vi "SignalViewer.vi"() -> ()   [LabVIEW 2014]
uses:
  <vilib>/Analysis/3filter.llb/Filter Passband Type.ctl
  <vilib>/Analysis/3filter.llb/Filter Structure Type.ctl
  <vilib>/event_ctls.llb/eventvkey.ctl
  <vilib>/Utility/miscctls.llb/LVPositionTypeDef.ctl
  <vilib>/Utility/miscctls.llb/LVKeyTypeDef.ctl
  <vilib>/imath/engines/lvmath/Plug In/_Char/NIMS_CH_character datatype.ctl
  <vilib>/Analysis/2dsp.llb/Decimate (single shot, DBL).vi
  <vilib>/Analysis/baseanly.llb/Mean (DBL).vi
  <vilib>/Analysis/3filter.llb/Savitzky-Golay Filter (DBL).vi
  <vilib>/Waveform/WDTOps.llb/WDT Waveform Duration DBL.vi
  <vilib>/Utility/file.llb/Write To Spreadsheet File (string).vi
  <vilib>/Utility/file.llb/Read From Spreadsheet File (string).vi
  <vilib>/Waveform/WDTOps.llb/WDT Get Waveform Time Array DBL.vi
  <vilib>/Waveform/WDTOps.llb/WDT Scale Delta t DBL.vi
  <vilib>/Waveform/WDTOps.llb/WDT Get Waveform Subset DBL.vi
  <vilib>/measure/matone.llb/Extract Single Tone Information 1 Chan.vi
  <vilib>/Analysis/3filter.llb/Zero Phase Filter (Cascade, DBL).vi
  <vilib>/addons/Time Frequency Analysis/Spectrogram.llb/TFA STFT Spectrogram (Waveform).vi
  <vilib>/addons/Time Frequency Analysis/_control.llb/TFA Configure Spectrogram Indicator (Predefined Color Table).vi
  <vilib>/addons/Time Series Analysis/Correlation and Spectral Analysis.llb/TSA Welch (Waveform).vi
  <vilib>/imath/engines/lvmath2/RunTimeEngine/Managers/WorkSpace/UID Generator.vi
  <vilib>/imath/engines/lvmath2/RunTimeEngine/BuiltInFunctions/win_hamming/NIMS_win_hamming.vi
  <vilib>/imath/engines/lvmath2/RunTimeEngine/ErrorHandling/NIMS_Error From Error Code.vi
  <vilib>/imath/engines/lvmath2/RunTimeEngine/BuiltInFunctions/coherence/NIMS_coherence().vi
  <instcachedir>/0/NIMS_coherence()_7638C21039694BA7B313C9663B018448.lvgen/NIMS_coherence()_7638C21039694BA7B313C9663B018448_000.vi
  <vilib>/imath/engines/lvmath2/RunTimeEngine/ErrorHandling/NIMS_Create Error From Enums.vi
  <vilib>/imath/engines/lvmath2/RunTimeEngine/IndexRead/NIMS M(S).vi
  <instcachedir>/0/NIMS M(S)_B826C018497E4940AE96BD27B540B6FB.lvgen/NIMS M(S)_B826C018497E4940AE96BD27B540B6FB_000.vi
  <vilib>/imathl/engines/lvmath/Functions/Error Handling/Create Error.vi
  <vilib>/imath/engines/lvmath2/RunTimeEngine/BuiltInFunctions/crosspsd/NIMS_crosspsd().vi
  <instcachedir>/0/NIMS_crosspsd()_8F170A66E657497C8ED809E1A8C589EF.lvgen/NIMS_crosspsd()_8F170A66E657497C8ED809E1A8C589EF_000.vi
  <vilib>/imath/engines/lvmath2/RunTimeEngine/RunTimeType/NIMS_RunTimeType_From StrictType (excl LVString).vi
  <instcachedir>/0/NIMS_RunTimeType_From StrictType (excl LVString)_15A5391EEA9C4AACB9955AC755B83D29.lvgen/NIMS_RunTimeType_From StrictType (excl LVString)_15A5391EEA9C4AACB9955AC755B83D29_000.vi
  <vilib>/imath/engines/lvmath2/RunTimeEngine/LocalVariableDefStatement/MC_LocalVariableDefStatement_Display.vi
  <vilib>/imath/engines/lvmath2/RunTimeEngine/BuiltInFunctions/conjugate/NIMS_conjugate(Complex).vi
  <instcachedir>/0/NIMS_conjugate(Complex)_151E186CA54B4853A0120BB0A667D86E.lvgen/NIMS_conjugate(Complex)_151E186CA54B4853A0120BB0A667D86E_001.vi
  <vilib>/imath/engines/lvmath2/RunTimeEngine/BuiltInFunctions/imag/NIMS_imag(Complex).vi
  <instcachedir>/0/NIMS_imag(Complex)_3180D40D00C843A49C2B33397F857BF3.lvgen/NIMS_imag(Complex)_3180D40D00C843A49C2B33397F857BF3_002.vi
  <vilib>/imath/engines/lvmath2/RunTimeEngine/BuiltInFunctions/angle/NIMS_angle.vi
  <instcachedir>/0/NIMS_angle_6DDAE2BD99E0421EB990B6436E94D88F.lvgen/NIMS_angle_6DDAE2BD99E0421EB990B6436E94D88F_002.vi
  <vilib>/imath/engines/lvmath2/RunTimeEngine/BuiltInFunctions/rad_to_deg/NIMS_rad_to_deg.vi
  <instcachedir>/0/NIMS_rad_to_deg_A39AFCDDC8C049FCADAAB7FC30B9F5AA.lvgen/NIMS_rad_to_deg_A39AFCDDC8C049FCADAAB7FC30B9F5AA_001.vi
  <vilib>/imath/engines/lvmath2/RunTimeEngine/BuiltInFunctions/unwrapphase/NIMS_unwrapphase(M,M,I32).vi
  <vilib>/imath/engines/lvmath2/RunTimeEngine/BuiltInFunctions/abs/NIMS_abs(signed).vi
  <instcachedir>/0/NIMS_abs(signed)_C4FCB8E6058B49B797C7C8D53CA5F6EC.lvgen/NIMS_abs(signed)_C4FCB8E6058B49B797C7C8D53CA5F6EC_006.vi
  <vilib>/imath/engines/lvmath2/RunTimeEngine/NodeEndStatement/NIMS_NodeEndStatement_Get Vector.vi
  <instcachedir>/0/NIMS_NodeEndStatement_Get Vector_00D1625602D843AD9D7EC134A9EC13A2.lvgen/NIMS_NodeEndStatement_Get Vector_00D1625602D843AD9D7EC134A9EC13A2_001.vi
  <vilib>/imath/engines/lvmath/Functions/Error Handling/MergeErrorsWrapper.vi
  <vilib>/imath/engines/lvmath2/RunTimeEngine/Managers/SymbolTable/Clear UID.vi
  <vilib>/imath/engines/lvmath2/RunTimeEngine/NodeEndStatement/NIMS_NodeEndStatement_Output.vi
  <instcachedir>/0/NIMS_NodeEndStatement_Output_53EC0D466D134D7ABD903AC30B43404B.lvgen/NIMS_NodeEndStatement_Output_53EC0D466D134D7ABD903AC30B43404B_001.vi
  <instcachedir>/0/NIMS_NodeEndStatement_Output_53EC0D466D134D7ABD903AC30B43404B.lvgen/NIMS_NodeEndStatement_Output_53EC0D466D134D7ABD903AC30B43404B_005.vi
  <vilib>/imath/engines/lvmath2/RunTimeEngine/ErrorHandling/NIMS_Finalize Error.vi
  <vilib>/imath/engines/lvmath2/RunTimeEngine/BuiltInFunctions/psd_welch/NIMS_psd_welch().vi
  <instcachedir>/0/NIMS_psd_welch()_5616DAC80B234F9987AA290C647A4538.lvgen/NIMS_psd_welch()_5616DAC80B234F9987AA290C647A4538_000.vi
  <vilib>/imath/engines/lvmath2/RunTimeEngine/IndexRead/NIMS V(S).vi
  <instcachedir>/0/NIMS V(S)_0488751826AF41519A22953C041130DC.lvgen/NIMS V(S)_0488751826AF41519A22953C041130DC_000.vi
  <vilib>/addons/_Advanced Signal Processing/NI_AdvSigProcTSA.lvlib
  <vilib>/Analysis/NI_AALBase.lvlib
  <vilib>/addons/_Advanced Signal Processing/NI_AdvSigProcTFA.lvlib
  <vilib>/measure/NI_MAPro.lvlib
  <vilib>/imath/engines/lvmath2/RunTimeEngine/Managers/SymbolTable/NIMS_WorkSpace.lvlib
  <vilib>/Analysis/NI_AALPro.lvlib
panel:
  out "listOfProfiles":path[](array[path])
  in  "write":bool
  in  "XY":bool
  in  "picker":i32(ring) items=["AllPlots", "13.06.17\\_0005#2_dt=2.40E-6orig", "13.06.17\\_0005#4_dt=2.40E-6orig", "13.06.17\\_0005#6_dt=2.40E-6orig", "13.06.17\\_0005#10_dt=2.40E-6orig"]
  in  "step, ms":dbl=1.0
  in  "howmany":u32=10 min=1
  in  "points":bool
  in  "clear":bool
  in  "scale fit":bool
  in  "path-name":bool=TRUE
  in  "show legend":bool
  in  "data info template":T1={"data path"="", "ADCintercadr_s"=1.0, "data info"={"use or not *.info.txt?"=0, "probe name"="NaN", "signal type"="NaN", "Unit"="NaN", "variable"="NaN", "attenuation factor"=1.0, "amplification factor"=1.0, "extracoef#1"=1.0, "extracoef#2"=1.0, "U cascade, kV"="NaN", "probe area, cm2"=1.0, "plasma, a.m.u."=1.0}, "channel_name"="", "channels_in_file"=0, "LastModified"=""}
  out "allinfos":T2(array[cluster])
  in  "0-color":u32(colorbox)=4456703
  in  "\"0\" line":bool
  in  "zero drift control":T3={"start zero, ms"=1.0, "duration of zero,ms"=1.0, "'0',\nms"=FALSE} {"start zero, ms" min=0.002400000058593751 max=49.996801220625024; "duration of zero,ms" min=0.002400000058593751 max=49.996801220625024}
  in  "autopen":cluster{"howmany":i16, "auto/man.":bool}={"howmany"=1, "auto/man."=FALSE} {"howmany" min=1}
  in  "show all":bool
  in  "cleararray":bool
  in  "regime":u16(ring) items=["data", "spectfilt", "preprocessed", "triple probe"]
  in  "open":bool
  in  "applyInfo":bool
  in  "setInfo":bool
  in  "writedat":bool
  out "spectrogram array":dbl[][][](array[numeric])
  in  "scalefit2":bool
  out "chan.in.files":i16[](array[numeric])
  in  "curs.":bool
  in  "curs.0":bool
  out "cursors":T4 {"Y1" format="%#.7f"; "X1" format="%#.7f"; "Y" format="%#.7f"; "X" format="%#.7f"}
  in  "EX":bool
  in  "width":i16 min=0 max=5 step=1
  in  "aver.\ncolor":u32(colorbox)=16711680
  in  "smooth":u16(ring) items=["origin"=0, "orig&med"=5, "orig-med"=6, "orig&poly"=1, "orig-poly"=3, "polynom"=2, "median"=4]
  in  "polyn.\norder":i32=1 min=1
  in  "wind.,\nms":dbl=1.0 min=0.004800000117187502 max=24.998400610312512
  out "nextfile":bool
  out "return pressed?":bool
  out "recalculate?":bool
  in  "tripleProbeSetting":T5={"Isat"=0, "Vfl"=0, "V+"=0, "a=1/ln2"=1.44, "Vfl*"=1.0, "[V+]*"=1.0, "Te*"=2.5, "/Rn(ohm)"=1.0, "/amplif"=1.0, "Spr, cm^2"=0.07, "plasma, a.m.u"=1.0, "Ne*10^x"=11.0} {"Ne*10^x" min=1.0 max=20.0 step=1.0; "V+" items=["14.06.17\\_0001=t0.000000-0.050000#2", "14.06.17\\_0001=t0.000000-0.050000#4", "14.06.17\\_0001=t0.000000-0.050000#6", "14.06.17\\_0002=t0.000000-0.050000#2", "14.06.17\\_0002=t0.000000-0.050000#4", "14.06.17\\_0002=t0.000000-0.050000#6", "14.06.17\\_0003=t0.000000-0.050000#2", "14.06.17\\_0003=t0.000000-0.050000#4", "14.06.17\\_0003=t0.000000-0.050000#6", "14.06.17\\_0004=t0.000000-0.050000#2", "14.06.17\\_0004=t0.000000-0.050000#4", "14.06.17\\_0004=t0.000000-0.050000#6", "14.06.17\\_0005=t0.000000-0.050000#2", "14.06.17\\_0005=t0.000000-0.050000#4", "14.06.17\\_0005=t0.000000-0.050000#6"]; "Vfl" items=["14.06.17\\_0001=t0.000000-0.050000#2", "14.06.17\\_0001=t0.000000-0.050000#4", "14.06.17\\_0001=t0.000000-0.050000#6", "14.06.17\\_0002=t0.000000-0.050000#2", "14.06.17\\_0002=t0.000000-0.050000#4", "14.06.17\\_0002=t0.000000-0.050000#6", "14.06.17\\_0003=t0.000000-0.050000#2", "14.06.17\\_0003=t0.000000-0.050000#4", "14.06.17\\_0003=t0.000000-0.050000#6", "14.06.17\\_0004=t0.000000-0.050000#2", "14.06.17\\_0004=t0.000000-0.050000#4", "14.06.17\\_0004=t0.000000-0.050000#6", "14.06.17\\_0005=t0.000000-0.050000#2", "14.06.17\\_0005=t0.000000-0.050000#4", "14.06.17\\_0005=t0.000000-0.050000#6"]; "Isat" items=["14.06.17\\_0001=t0.000000-0.050000#2", "14.06.17\\_0001=t0.000000-0.050000#4", "14.06.17\\_0001=t0.000000-0.050000#6", "14.06.17\\_0002=t0.000000-0.050000#2", "14.06.17\\_0002=t0.000000-0.050000#4", "14.06.17\\_0002=t0.000000-0.050000#6", "14.06.17\\_0003=t0.000000-0.050000#2", "14.06.17\\_0003=t0.000000-0.050000#4", "14.06.17\\_0003=t0.000000-0.050000#6", "14.06.17\\_0004=t0.000000-0.050000#2", "14.06.17\\_0004=t0.000000-0.050000#4", "14.06.17\\_0004=t0.000000-0.050000#6", "14.06.17\\_0005=t0.000000-0.050000#2", "14.06.17\\_0005=t0.000000-0.050000#4", "14.06.17\\_0005=t0.000000-0.050000#6"]}
  in  "inpcontrclaster":T6={"showwhat"={"total\nplots"=4, "show\nplots"=100, "show one/all"=FALSE, "ch#"=1, "visible\nplots"=4, "main loop\nwait, ms"=-1, "Y shift"=0.0, "txt rate,kHz"=625.0, "AxisX"=1, "X shift,ms"=0.0}, "inp.control"=[{"dataname"=0, "X-shift, ms"=0.0, "Y-shift"=0.0, "width"=0, "Color"=0, "visible"=TRUE, "multiplic."=1.0}, {"dataname"=0, "X-shift, ms"=0.0, "Y-shift"=0.0, "width"=0, "Color"=128, "visible"=TRUE, "multiplic."=1.0}, {"dataname"=0, "X-shift, ms"=0.0, "Y-shift"=0.0, "width"=0, "Color"=16711680, "visible"=TRUE, "multiplic."=1.0}, {"dataname"=0, "X-shift, ms"=0.0, "Y-shift"=0.0, "width"=0, "Color"=65280, "visible"=TRUE, "multiplic."=1.0}], "factor"=0, "average"=FALSE, "decimate"=FALSE} {"factor" min=1; "inp.control"."multiplic." format="%_6g"; "inp.control"."width" min=0 max=5 step=1; "inp.control"."Y-shift" format="%.6f"; "inp.control"."dataname" items=["***", "_0005#2\\13.06.17", "_0005#4\\13.06.17", "_0005#6\\13.06.17", "_0005#10\\13.06.17"]; "showwhat"."AxisX" items=["index", "time,s", "time,ms"]; "showwhat"."main loop\nwait, ms" min=-1 step=1; "showwhat"."visible\nplots" min=1 max=3; "showwhat"."ch#" min=0 max=4; "showwhat"."show\nplots" min=1; "showwhat"."total\nplots" min=1 max=3}
  in  "preproc.settings":T7={"select1"=0, "select2"=0, "FFT Window info"={"Window"=2, "Length"=128, "Overlap (%)"=50.0, "log/lin"=FALSE}, "dist.,cm"=0.3, "PowerScale 2D"=1.0, "Plot.Line Width"=3, "spectrogram\nsampling inf"={"time steps"=-1, "frequency bins"=512}, "dB on?"=FALSE, "spctrgr.color"=0, "spctrgrmWhich"=0, "autoscale"=TRUE, "max.freq,Hz"=0.0, "maxFreqSet"=FALSE} {"spctrgrmWhich" items=["14.06.17\\_0010=t0.000000-0.050000#2", "14.06.17\\_0010=t0.000000-0.050000#4", "14.06.17\\_0010=t0.000000-0.050000#6", "14.06.17\\_0010=t0.000000-0.050000#10"]; "spctrgr.color" items=["Rainbow", "Inverse gray", "Gray"]; "Plot.Line Width" max=5; "select2" items=["coherence", "crosspsd", "phase", "phaseDegrees", "Wavenum", "Flux(nv)"]; "PowerScale 2D" format="%#_6e"; "select1" items=["preproc.data", "crossfunct.", "autopsd", "spctrgrm"]; "FFT Window info"."Window" items=["None ", "Hanning", "Hamming", "Blackman-Harris", "Exact Blackman", "Blackman", "Flat Top", "4 Term B-Harris ", "7 Term B-Harris", "Low Sidelobe"]}
  out "triple probe":waveform(dbl)[](graph)
  out "spctrgrmClaster":T8 {"X" format="%#.6f"}
  out "scale info":variant
  out "observeddir":T9
  out "cut.filtered":waveform(dbl)[](graph)
  out "source":T10
  out "data cut":T11
  in  "spectr.filt.":enum32{"Page 1"}(tab)
  out "singletoneresult":waveform(dbl)(graph)
  in  "lin/log":u8(ring) items=["lin", "log"]
  in  "channel":i32(ring) items=["14.06.17\\_0010=t0.000000-0.050000#2", "14.06.17\\_0010=t0.000000-0.050000#4", "14.06.17\\_0010=t0.000000-0.050000#6", "14.06.17\\_0010=t0.000000-0.050000#10"]
  in  "singletonecontroll":T12={"advanced search"={"approx.freq."=-1.0, "search(+/-%)"=5.0}, "remove\ntone"=FALSE} {"advanced search"."search(+/-%)" format="%0.2p"; "advanced search"."approx.freq." format="%0.2p"}
  out "singletone":T13 {"det. phase (deg)" format="%.2p"; "detect.freq.,Hz" format="%.4e"; "detected ampl." format="%#.4e"}
  in  "bandstop":T16={"order"=4, "filter type"=enum."Bandstop", "filter structure option"=10, "apply\nfilter"=FALSE} {"filter structure option" items=["IIR 2nd Order"=0, "IIR 4th Order"=1, "Auto Select"=10]}
  in  "export mode":T17(ring)=enum."residual signal"
  in  "show":bool
  in  "time-freq. sampling info":cluster{"time steps":i32, "freq.bins":i32}={"time steps"=-1, "freq.bins"=1024}
  in  "spectrogam window info":cluster{"type":i32, "length":i32}={"type"=2, "length"=-1} {"type" items=["None ", "Hanning", "Hamming", "Blackman-Harris", "Exact Blackman", "Blackman", "Flat Top", "4 Term B-Harris ", "7 Term B-Harris", "Low Sidelobe", "Gaussian"]}
  in  "color table":u16(ring) items=["Rainbow", "Inverse gray", "Gray"]
  in  "fit":bool=TRUE
  in  "dB on?":bool
  out "PSD":cluster{"f0":dbl, "df":dbl, "S(f)":dbl[]}(graph)={"f0"=0.0, "df"=2441.40625, "S(f)"=[]}
  in  "window info":T18={"window"=2, "length"=64, "overlap (%)"=50.0} {"window" items=["None ", "Hanning", "Hamming", "Blackman-Harris", "Exact Blackman", "Blackman", "Flat Top", "4 Term B-Harris ", "7 Term B-Harris", "Low Sidelobe"]}
  in  "freq.bins":i32=1024
  out "Spectrogram":dbl[][](graph)
  in  "param.table":T19={"data info manual input sample"=[["11_00_19", "2", "VG1#1", "LP_biasing", "10.25", "1", "1", "162", "1", "5,6", "0.07", "1"], ["=", "4", "VG1#2", "LP_current", "10.25", "1", "1", "300", "1", "5,6", "0.07", "1"], ["11_00_44", "2", "VG1#1", "LP_biasing", "10.25", "1", "1", "162", "1", "5,6", "0.07", "1"], ["=", "4", "VG1#2", "LP_current", "10.25", "1", "1", "300", "1", "5,6", "0.07", "1"]], "data info manual input"=[["11", "7", "VG8", "V", "10.25", "1", "1", "", "", "", "0.049", "1"], ["=", "0", "VG8", "I", "10.25", "1", "1", "", "", "", "0.049", "1"], ["=", "10", "VG8", "V", "10.25", "1", "1", "", "", "", "0.049", "1"], ["=", "0", "VG8", "I", "10.25", "1", "1", "", "", "", "0.049", "1"]], "press after parram.input"=FALSE}
  out "data view":waveform(dbl)[](graph) caption="ADC data"
  # "Te=([V+]-[Vfl])*a"
  # "Vpl=Vfl+d*Te"
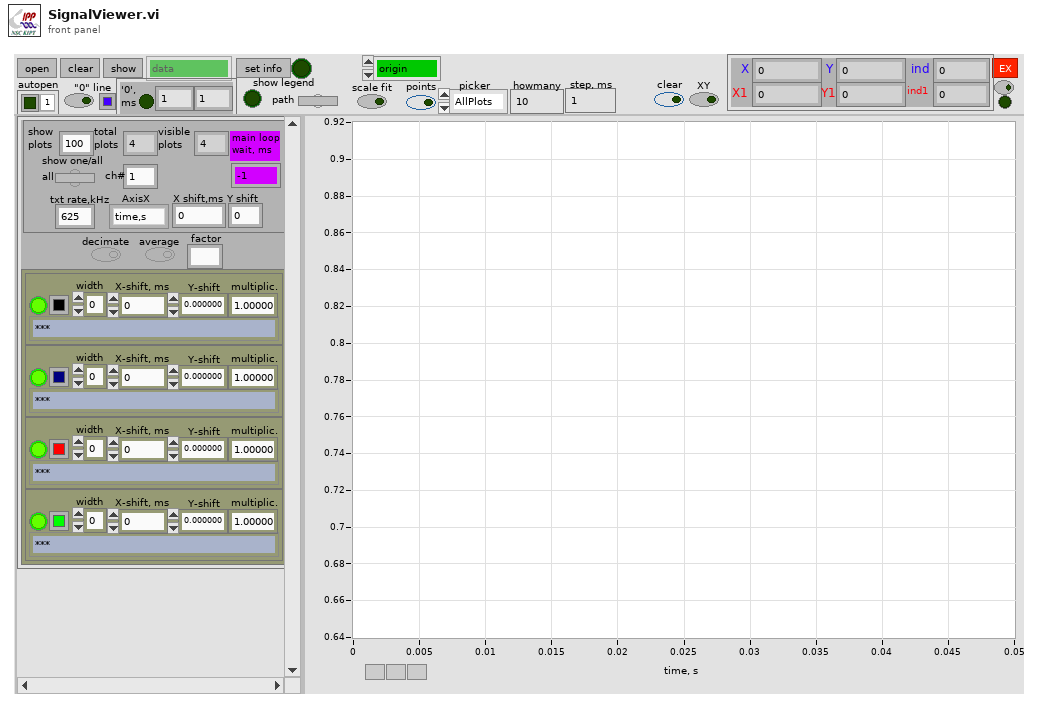
[diagram p1: front panel]
types:
  T1 = cluster{"data path":string, "ADCintercadr_s":dbl, "data info":cluster{"use or not *.info.txt?":i16, "probe name":string, "signal type":string, "Unit":string, "variable":string, "attenuation factor":dbl, "amplification factor":dbl, "extracoef#1":dbl, "extracoef#2":dbl, "U cascade, kV":string, "probe area, cm2":dbl, "plasma, a.m.u.":dbl}, "channel_name":string, "channels_in_file":i32, "LastModified":string}
  T2 = cluster{"data path":string, "ADCintercadr_s":dbl, "data info":cluster{"use or not *.info.txt?":i16, "probe name":string, "signal type":string, "Unit":string, "variable":string, "attenuation factor":dbl, "amplification factor":dbl, "extracoef#1":dbl, "extracoef#2":dbl, "U cascade, kV":string, "probe area, cm2":dbl, "plasma, a.m.u.":dbl}, "channel_name":string, "channels_in_file":i32, "LastModified":string}[]
  T3 = cluster{"start zero, ms":dbl, "duration of zero,ms":dbl, "'0',\nms":bool}
  T4 = cluster{"X":dbl, "Y":dbl, "ind":i32, "X1":dbl, "Y1":dbl, "ind1":i32}
  T5 = cluster{"Isat":u16, "Vfl":u16, "V+":u16, "a=1/ln2":dbl, "Vfl*":dbl, "[V+]*":dbl, "Te*":dbl, "/Rn(ohm)":dbl, "/amplif":dbl, "Spr, cm^2":dbl, "plasma, a.m.u":dbl, "Ne*10^x":dbl}
  T6 = cluster{"showwhat":cluster{"total\nplots":i16, "show\nplots":i16, "show one/all":bool, "ch#":i32, "visible\nplots":i16, "main loop\nwait, ms":i32, "Y shift":dbl, "txt rate,kHz":dbl, "AxisX":u16, "X shift,ms":dbl}, "inp.control":cluster{"dataname":u16, "X-shift, ms":dbl, "Y-shift":dbl, "width":i16, "Color":u32, "visible":bool, "multiplic.":dbl}[], "factor":i32, "average":bool, "decimate":bool}
  T7 = cluster{"select1":u16, "select2":u16, "FFT Window info":cluster{"Window":u16, "Length":i32, "Overlap (%)":dbl, "log/lin":bool}, "dist.,cm":dbl, "PowerScale 2D":dbl, "Plot.Line Width":u8, "spectrogram\nsampling inf":cluster{"time steps":i32, "frequency bins":i32}, "dB on?":bool, "spctrgr.color":u16, "spctrgrmWhich":u16, "autoscale":bool, "max.freq,Hz":dbl, "maxFreqSet":bool}
  T8 = cluster{" time info":cluster{"time offset":dbl, "time multipl.":dbl}, "frequency info":cluster{"freq. offset":dbl, "freq. multipl.":dbl}, "Spectrogram":dbl[][], "frequency marginal integral":cluster{"freq. offset":dbl, "freq. multipl.":dbl, "Value":dbl[]}, "time marginal integral ":cluster{"freq. offset":dbl, "freq. multipl.":dbl, "Value":dbl[]}, "instantaneous PSD":cluster{"freq. offset":dbl, "freq. multipl.":dbl, "Value":dbl[]}, "X":dbl}
  T9 = cluster{"last mod":timestamp, "stripped path":path}
  T10 = cluster{"data path":string[], "data":waveform(dbl)[]}
  T11 = cluster{"data offset array":dbl[], "data cut array":waveform(dbl)[], "data lables":string[], "short data lables":string[]}
  T12 = cluster{"advanced search":cluster{"approx.freq.":dbl, "search(+/-%)":dbl}, "remove\ntone":bool}
  T13 = cluster{"detect.freq.,Hz":dbl, "detected ampl.":dbl, "det. phase (deg)":dbl}
  T14 = typedef "NI_AALBase.lvlib/Filter Passband Type.ctl" = enum32{"Lowpass", "Highpass", "Bandpass", "Bandstop"}
  T15 = typedef "NI_AALBase.lvlib/Filter Structure Type.ctl" = u16
  T16 = cluster{"order":i32, "filter type":T14, "filter structure option":T15, "apply\nfilter":bool}
  T17 = enum32{"none", "input signal", "detected signal", "residual signal"}
  T18 = cluster{"window":u16, "length":i32, "overlap (%)":dbl}
  T19 = cluster{"data info manual input sample":string[][], "data info manual input":string[][], "press after parram.input":bool}
  T20 = typedef "eventvkey.ctl" = enum16{"ASCII", "Enter", "Return", "Shift", "Ctrl", "Alt", "Cmd", "Opt", "Caps", "NumLock", "Clear", "Break", "Up", "Down", "Left", "Right", "Insert", "Delete", "Home", "End", "PageUp", "PageDown", "Escape", "Help", "Pause", "ScrollLock", "F1", "F2", "F3", "F4", "F5", "F6", "F7", "F8", "F9", "F10", "F11", "F12", "F13", "F14", "F15", "F16", "F17", "F18", "F19", "F20", "F21", "F22", "F23", "F24", "Play", "VolumeUp", "VolumeDown", "Mute", "Two Byte Char"}
  T21 = typedef "LVPositionTypeDef.ctl" = cluster{"Left":i32, "Top":i32}
  T22 = enum8{"Enabled", "Disabled", "Disabled and Grayed Out"}
  T23 = cluster{"dataname":u16, "X-shift":i32, "Y-shift":dbl, "width":i16, "Color":u32, "visible":bool, "multiplic.":dbl}
  T24 = typedef "LVKeyTypeDef.ctl" = cluster{"Focus":bool, "Control":bool, "Shift":bool, "Key":string}
  T25 = cluster{"Name":string, "Color":u32, "Style":u8, "Point Style":u8, "Name Visible":bool, "Allow Drag":bool, "Cursor Mode":u32, "Plot":i32, "Index":i32, "Position":cluster{"X":dbl, "Y":dbl}, "X Scale":u32, "Y Scale":u32, "Watch Plots":i32[], "Watch All Plots":bool, "Plot Area":i32, "Label Offset":cluster{"X":dbl, "Y":dbl}}
  T26 = typedef "NIMS_CH_character datatype.ctl" = cluster{"Numeric":u8}
  T27 = typedef "LVCursorListTypeDef.ctl" = cluster{"Name":string, "Color":u32, "Style":u8, "Point Style":u8, "Name Visible":bool, "Allow Drag":bool, "Cursor Mode":u32, "Plot":i32, "Index":i32, "Position":cluster{"X":dbl, "Y":dbl}, "X Scale":u32, "Y Scale":u32, "Watch Plots":i32[], "Watch All Plots":bool, "Plot Area":i32, "Label Offset":cluster{"X":dbl, "Y":dbl}}[]
  T28 = cluster{"dataname":u16, "X-shift":i32, "Y-shift":dbl, "width":i16, "Color":u32, "visible":bool, "multiplic.":dbl}[]
  T29 = cluster{"total\nplots":i16, "show\nplots":i16, "show one/all":bool, "ch#":i32, "visible\nplots":i16, "main loop\nwait, ms":i32, "Y shift":dbl, "txt rate,kHz":dbl, "AxisX":u16, "X shift,ms":dbl}
  T30 = cluster{"dataname":u16, "X-shift, ms":dbl, "Y-shift":dbl, "width":i16, "Color":u32, "visible":bool, "multiplic.":dbl}[]
  T31 = cluster{"dataname":u16, "X-shift, ms":dbl, "Y-shift":dbl, "width":i16, "Color":u32, "visible":bool, "multiplic.":dbl}
  T32 = typedef "imagedata.ctl" = cluster{"image type":i32, "image depth":i32, "image":u8[], "mask":u8[], "colors":u32[], "Rectangle":cluster{"left":i16, "top":i16, "right":i16, "bottom":i16}}
  T33 = cluster{"show legend":bool, "path-name":bool, "aver.\ncolor":u32, "width":i16}
  T34 = cluster{"use or not *.info.txt?":i16, "probe name":string, "signal type":string, "Unit":string, "variable":string, "attenuation factor":dbl, "amplification factor":dbl, "extracoef#1":dbl, "extracoef#2":dbl, "U cascade, kV":string, "probe area, cm2":dbl, "plasma, a.m.u.":dbl}
  T35 = typedef "LVPointDoubleTypeDef.ctl" = cluster{"Cursor X":dbl, "Cursor Y":dbl}
  T36 = typedef "LVRangeTypeDef.ctl" = cluster{"Minimum":dbl, "Maximum":dbl, "Increment":dbl, "Minor Increment":dbl, "Start":dbl}
  T37 = typedef "LVPoint32TypeDef.ctl" = cluster{"Horizontal":i32, "Vertical":i32}
  T38 = cluster{"Shift":bool, "Ctrl":bool, "Alt":bool, "Cmd":bool, "Opt":bool}
  T39 = cluster{"filter structure":enum32{"IIR 2nd Order", "IIR 4th Order"}, "Reverse Coefficients":dbl[], "Forward Coefficients":dbl[]}
  T40 = cluster{"exported time signal":waveform(dbl), "exported spectrum (dB)":cluster{"f0":dbl, "df":dbl, "dB Spectrum (Hann)":dbl[]}}
  T41 = cluster{"detected frequency":dbl, "detected amplitude":dbl, "detected phase (deg)":dbl}
  T42 = cluster{"Window":u16, "Length":i32, "Overlap (%)":dbl, "log/lin":bool}
  T43 = cluster{"frequency offset":dbl, "frequency multiplier":dbl}
  T44 = cluster{"time offset":dbl, "time multiplier":dbl}
  T45 = cluster{"frequency offset":dbl, "frequency multiplier":dbl, "Value":dbl[]}
  T46 = cluster{"time info":cluster{"time offset":dbl, "time multiplier":dbl}, "frequency info":cluster{"frequency offset":dbl, "frequency multiplier":dbl}, "Value":dbl[][], "frequency marginal integral":cluster{"f0":dbl, "df":dbl, "spectrum":dbl[]}, "time marginal integral":cluster{"t0":dbl, "dt":dbl, "power":dbl[]}, cluster{"frequency offset":dbl, "frequency multiplier":dbl, "Value":dbl[]}, "Cursor.Cursor X":dbl}
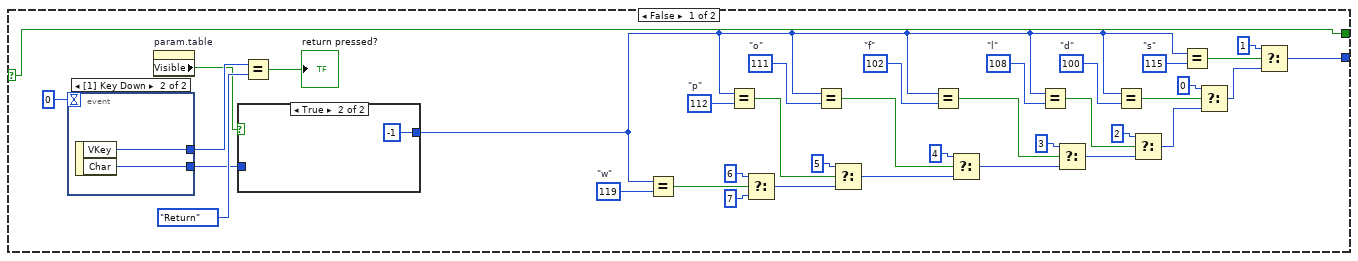
[diagram p3: hidden frame]
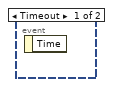
[diagram p5: hidden frame]
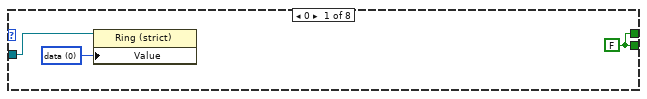
[diagram p6: hidden frame]
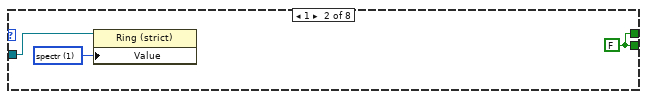
[diagram p7: hidden frame]
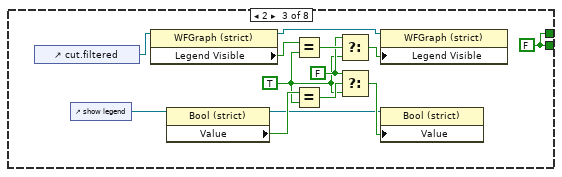
[diagram p8: hidden frame]
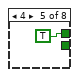
[diagram p9: hidden frame]
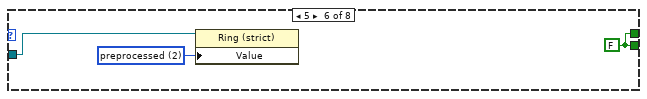
[diagram p10: hidden frame]
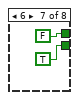
[diagram p11: hidden frame]
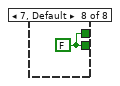
[diagram p12: hidden frame]
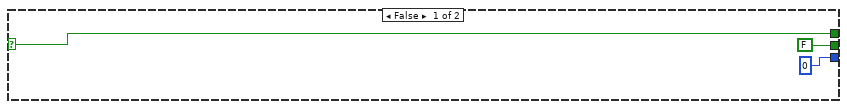
[diagram p14: hidden frame]
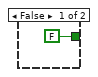
[diagram p16: hidden frame]
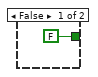
[diagram p18: hidden frame]
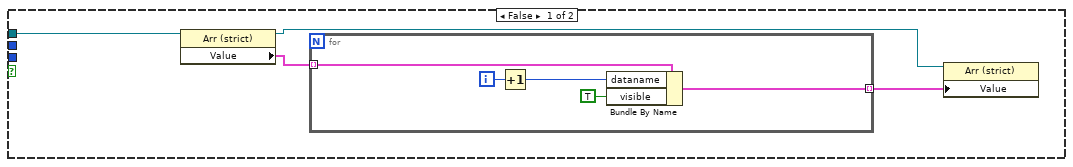
[diagram p19: hidden frame]
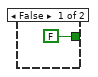
[diagram p20: hidden frame]
diagram:
  n1 = while {
    i -> [w3]
    stop <- FALSE stop-if-true
    n2 = flat-sequence {
      tunnel: w3 -> [w13]
      tunnel: [w13] -> w1
      tunnel: [w16] -> w2
      tunnel: w1 -> [w17]
      tunnel: [w81] -> w4
      tunnel: w2 -> [w80]
      tunnel: [w132] -> w8
      tunnel: [w139] -> w7
      tunnel: [w140] -> w6
      tunnel: [w137] -> w5
      tunnel: w4 -> [w130]
      tunnel: w8 -> [w260]
      tunnel: w7 -> [w259]
      tunnel: w6 -> [w258]
      tunnel: w5 -> [w257]
      frame #0 {
        n3 = invoke on="data view" class="WFGraph (strict)" method="ForceRedraw"() -> ()  [unwired: 3 in, 3 out]
        n4 = Unbundle By Name("inpcontrclaster") -> ("showwhat.main loop\nwait, ms"=w11:i32)
        n5 = control-ref of="This VI"() -> (w12:refnum<vi>)
        n6 = Wait For Front Panel Activity(1:w11, 2:w12) -> ()  [unwired: 1 in, 1 out]
      }
      frame #1 {
        n7 = Equal To 0?(x=w17) -> (x = 0?=w18:bool)
        n8 = case shown="True" w18 {
          selector: w18 -> [w24 w66]
          tunnel: [w37 7 ("f")] -> w16
          tunnel: [w24 w66] -> w14
          frame False {
            w31 = i16 119  # "w"
            w59 = i16 112  # "p"
            w56 = i16 111  # "o"
            w51 = i16 102  # "f"
            w47 = i16 108  # "l"
            w42 = i16 100  # "d"
            w39 = i16 115  # "s"
            n9 = event shown="[1] Key Down" {
              selector: _ -> [_ _]
              dyn-events: _ -> [_ _]
              timeout: 0 -> [_ _]
              tunnel: [_ w64] -> w26
              tunnel: [_ w63] -> w28
              event Timeout {
                n10 = event-data() -> ()  [unwired: 1 in, 1 out]
              }
              event Key Down {
                n11 = event-data() -> ("VKey"=w63:T20, "Char"=w64:i16)  [unwired: 1 in]
              }
            }
            n12 = property on="param.table" class="Clust"() -> ("Visible"=w27:bool)  [unwired: 2 in, 2 out]
            n13 = case shown="True" w27 {
              tunnel: w26 -> [w61 _]
              tunnel: [w61 -1] -> w25
              frame False {
              }
              frame True {
              }
            }
            n14 = Equal?(x=w28, y=eventvkey."Return") -> (x = y?=→"return pressed?":bool)
            n15 = Equal?(x=w25, y=w31) -> (x = y?=w33:bool)
            n16 = Equal?(x=w25, y=w59) -> (x = y?=w36:bool)
            n17 = Select(t=6 ("f"), s=w33, f=7) -> (s? t:f=w34:i32)
            n18 = Equal?(x=w25, y=w56) -> (x = y?=w57:bool)
            n19 = Select(t=5 ("f"), s=w36, f=w34) -> (s? t:f=w60:i32)
            n20 = Equal?(x=w25, y=w51) -> (x = y?=w50:bool)
            n21 = Select(t=4 ("f"), s=w57, f=w60) -> (s? t:f=w55:i32)
            n22 = Equal?(x=w25, y=w47) -> (x = y?=w46:bool)
            n23 = Select(t=3 ("f"), s=w50, f=w55) -> (s? t:f=w53:i32)
            n24 = Equal?(x=w25, y=w42) -> (x = y?=w43:bool)
            n25 = Select(t=2 ("f"), s=w46, f=w53) -> (s? t:f=w48:i32)
            n26 = Equal?(x=w25, y=w39) -> (x = y?=w40:bool)
            n27 = Select(t=0 ("f"), s=w43, f=w48) -> (s? t:f=w45:i32)
            n28 = Select(t=1, s=w40, f=w45) -> (s? t:f=w37:i32)
          }
          frame True {
            n29 = call "Display Message to User"("Enable"=FALSE) -> ()  [unwired: 9 in, 2 out]
            n30 = property on="inpcontrclaster" class="Clust (strict)"("Position"=T21 {"Left"=0, "Top"=0}) -> ()  [unwired: 2 in, 2 out]
            n31 = property on="regime" class="Ring (strict)"("DisabledEnum"=T22."Disabled and Grayed Out" ("Disabled")) -> (error out=w78:errorcluster)  [unwired: 2 in, 1 out]
            n32 = invoke on="regime" class="Ring (strict)" method="Reinit To Default"(error in=w78) -> (error out=w76:errorcluster)  [unwired: 2 in, 2 out]
            n33 = invoke on="cut.filtered" class="WFGraph (strict)" method="Reinit To Default"(error in=w76) -> (error out=w72:errorcluster)  [unwired: 2 in, 2 out]
            n34 = invoke on="data view" class="WFGraph (strict)" method="Reinit To Default"(error in=w72) -> (error out=w71:errorcluster)  [unwired: 2 in, 2 out]
            n35 = invoke on="data view" class="WFGraph (strict)" method="ForceRedraw"(error in=w71) -> (error out=w70:errorcluster)  [unwired: 2 in, 2 out]
            n36 = property on="Splitter 3" class="Splitter"(error in=w70, "Position"=1 ("Splitter Position")) -> (error out=w73:errorcluster)  [unwired: 1 in, 1 out]
            n37 = invoke on="smooth" class="Ring (strict)" method="Reinit To Default"(error in=w73) -> (error out=w68:errorcluster)  [unwired: 2 in, 2 out]
            n38 = property on="auto/man." class="Bool (strict)"(error in=w68, "Value"=FALSE) -> ()  [unwired: 1 in, 2 out]
          }
        }
        n39 = control-ref of="data view"() -> (w15:refnum<vi>)
        n40 = case shown="True" w14 {
          tunnel: w15 -> [_ w19]
          frame False {
          }
          frame True {
            n41 = property on="Property Node" class="WFGraph (strict)"(reference=w19) -> (reference out=w20:refnum<vi>, "CrsrList"=w23:T27)  [unwired: 1 in, 1 out]
            n42 = Array Subset(array=w23, length=3) -> (w21:T27)  [unwired: 1 in]
            n43 = property on="Property Node" class="WFGraph (strict)"(reference=w20, "CrsrList"=w21) -> ()  [unwired: 1 in, 2 out]
          }
        }
      }
      frame #2 {
        n44 = control-ref of="regime"() -> (w82:refnum<vi>)
        n45 = case shown="3" w80 {
          tunnel: w82 -> [w85 w88 _ _ _ w119 _ _]
          tunnel: [w83 w86 w89 w102 TRUE ("Value") w117 FALSE ("Value") w122] -> w81
          tunnel: [w83 w86 w89 w102 _ w117 TRUE ("writedat") w122] -> w79
          frame 0 {
            w83 = FALSE ("Value")
            w84 = u16 0 items=["data", "spectr", "preprocessed"] ("regime")
            n46 = property on="Property Node" class="Ring (strict)"(reference=w85, "Value"=w84) -> ()  [unwired: 1 in, 2 out]
          }
          frame 1 {
            w86 = FALSE ("Value")
            w87 = u16 1 items=["data", "spectr", "preprocessed"] ("regime")
            n47 = property on="Property Node" class="Ring (strict)"(reference=w88, "Value"=w87) -> ()  [unwired: 1 in, 2 out]
          }
          frame 2 {
            w89 = FALSE ("Value")
            w93 = FALSE ("t")
            w92 = TRUE ("Value")
            n48 = control-ref of="cut.filtered"() -> (w96:refnum<vi>)
            n49 = control-ref of="show legend"() -> (w101:refnum<vi>)
            n50 = property class="WFGraph (strict)"(reference=w96) -> (reference out=w91:refnum<vi>, "Legend Visible"=w94:bool)  [unwired: 1 in, 1 out]
            n51 = property class="Bool (strict)"(reference=w101) -> (reference out=w97:refnum<vi>, "Value"=w100:bool)  [unwired: 1 in, 1 out]
            n52 = Equal?(x=w94, y=w92) -> (x = y?=w95:bool)
            n53 = Equal?(x=w100, y=w92) -> (x = y?=w99:bool)
            n54 = Select(t=w93, s=w95, f=w92) -> (s? t:f=w90:bool)
            n55 = Select(t=w93, s=w99, f=w92) -> (s? t:f=w98:bool)
            n56 = property class="WFGraph (strict)"(reference=w91, "Legend Visible"=w90) -> ()  [unwired: 1 in, 2 out]
            n57 = property class="Bool (strict)"(reference=w97, "Value"=w98) -> ()  [unwired: 1 in, 2 out]
          }
          frame 3 {
            w102 = FALSE ("Value")
            w104 = u8 1 ("X Scale.Scale Fit")
            w105 = 0 ("Active X Scale")
            w107 = u8 1 ("X Scale.Scale Fit")
            w108 = 0 ("Active X Scale")
            w112 = 290 ("y")
            n58 = control-ref of="Splitter 2"() -> (w114:refnum<vi>)
            n59 = property class="Splitter"(reference=w114) -> (reference out=w110:refnum<vi>, "Position"=w113:i32)  [unwired: 1 in, 1 out]
            n60 = control-ref of="data view"() -> (w106:refnum<vi>)
            n61 = control-ref of="cut.filtered"() -> (w103:refnum<vi>)
            n62 = Equal?(x=w113, y=w112) -> (x = y?=w115:bool)
            n63 = property on="Property Node" class="WFGraph (strict)"(reference=w106, "ActXScl"=w108, "ActYScl"=w108, "XScale.ScaleFit"=w107, "YScale.ScaleFit"=w107) -> ()  [unwired: 1 in, 2 out]
            n64 = property on="Property Node" class="WFGraph (strict)"(reference=w103, "ActXScl"=w105, "ActYScl"=w105, "XScale.ScaleFit"=w104, "YScale.ScaleFit"=w104) -> ()  [unwired: 1 in, 2 out]
            n65 = Select(t=21 ("y"), s=w115, f=w112) -> (s? t:f=w111:i32)
            n66 = property on="Property Node" class="Splitter"(reference=w110, "Position"=w111) -> ()  [unwired: 1 in, 2 out]
          }
          frame 4 {
          }
          frame 5 {
            w117 = FALSE ("Value")
            w118 = u16 2 items=["data", "spectr", "preprocessed"] ("regime")
            n67 = property on="Property Node" class="Ring (strict)"(reference=w119, "Value"=w118) -> ()  [unwired: 1 in, 2 out]
          }
          frame 6 {
          }
          frame 7, Default {
            w122 = FALSE ("Value")
          }
        }
        n68 = property on="writedat" class="Bool (strict)"("Value"=w79) -> ()  [unwired: 2 in, 2 out]
      }
      frame #3 {
        n69 = Unbundle By Name("autopen") -> ("auto/man."=w135:bool)
        n70 = case shown="True" "EX" {
          selector: "EX" -> [_ w244]
          tunnel: [FALSE w244] -> w126
          frame False {
          }
          frame True {
            n71 = property on="data path" class="Arr (strict)"() -> ("Value"=w239:string[])  [unwired: 2 in, 2 out]
            n72 = invoke on="inp.control" class="Arr (strict)" method="Reinit To Default"() -> ()  [unwired: 3 in, 3 out]
            n73 = Index Array(array=w239) -> (element=w238:string)  [unwired: 1 in]
            n74 = String To Path(string=w238) -> (path=w237:path)
            n75 = Strip Path(path=w237) -> (stripped path=w235:path)  [unwired: 1 out]
            n76 = Strip Path(path=w235) -> (name=w236:string)  [unwired: 1 out]
            n77 = Concatenate Strings(w236, "tmp" ("name or relative path")) -> (w241:string)
            n78 = Build Path(base path=w235, name or relative path=w241) -> (appended path=w240:path)
            n79 = call <vilib>:"Check if File or Folder Exists.vi"("path"=w240) -> ("file or folder exists?"=w243:bool)  [unwired: 8 in, 2 out]
            n80 = case shown="True" w243 {
              tunnel: w240 -> [_ w246]
              frame False {
              }
              frame True {
                n81 = Delete(path (use dialog)=w246, entire hierarchy (F)=TRUE) -> ()  [unwired: 3 in, 3 out]
              }
            }
          }
        }
        n82 = case shown="True" w135 {
          selector: w135 -> [w218 w221]
          tunnel: [FALSE w223] -> w134
          tunnel: [0 2] -> w124
          tunnel: [w218 w221] -> w123
          frame False {
          }
          frame True {
            n83 = control-ref of="observeddir"() -> (w226:refnum<vi>)
            n84 = property class="Clust (strict)"(reference=w226) -> ("Value"=w227:T9)  [unwired: 1 in, 2 out]
            n85 = Unbundle By Name(w227) -> ("last mod"=w225:timestamp, "stripped path"=w224:path)
            n86 = File/Directory Info(path=w224) -> (size=w230:i64, last mod=w231:timestamp)  [unwired: 1 in, 5 out]
            n87 = Not Equal?(x=w225, y=w231) -> (x != y?=w223:bool)
            n88 = Equal?(x=w230, y=i64 0) -> (x = y?=w228:bool)
            n89 = case shown="True" w228 {
              frame False {
              }
              frame True {
                n90 = control-ref of="auto/man."() -> (w233:refnum<vi>)
                n91 = property class="Bool (strict)"(reference=w233, "Value"=FALSE) -> ()  [unwired: 1 in, 2 out]
              }
            }
          }
        }
        n92 = Quit LabVIEW(quit? (T)=w126) -> ()
        n93 = property on="main loop\nwait, ms" class="DigNum (strict)"("Blinking"=w123) -> ()  [unwired: 2 in, 2 out]
        n94 = property on="open" class="Bool"("DisabledEnum"=w124) -> ()  [unwired: 2 in, 2 out]
        n95 = Or(x="open", y=w134) -> (x .or. y?=w131:bool)
        n96 = Or(x=w131, y=w130) -> (x .or. y?=w127:bool)
        "nextfile" <- w127
        n97 = control-ref of="scalefit2"() -> (w128:refnum<vi>)
        n98 = control-ref of="Splitter"() -> (w138:refnum<vi>)
        n99 = control-ref of="Splitter 2"() -> (w141:refnum<vi>)
        n100 = property class="Bool (strict)"(reference=w128, "Value"=w127) -> ()  [unwired: 1 in, 2 out]
        n101 = case shown="True" w127 {
          tunnel: w141 -> [w142 w145]
          tunnel: [w142 w145] -> w140
          tunnel: [_ w165] -> w139
          tunnel: w138 -> [w143 w183]
          tunnel: [w143 w182] -> w137
          tunnel: "autopen" -> [_ w180]
          frame False {
          }
          frame True {
            w149 = u8 1 ("Response to Value Outside Limits:Maximum")
            w156 = 1000.0 ("y")
            n102 = control-ref of="data info template"() -> (w174:refnum<vi>)
            n103 = property class="Clust (strict)"(reference=w174) -> ("Value"=w175:T1)  [unwired: 1 in, 2 out]
            n104 = property on="txt rate,kHz" class="DigNum (strict)"() -> ("Value"=w161:dbl)  [unwired: 2 in, 2 out]
            n105 = call "DATAreader5.vi"("manual ADC rate, kHz"=w161, "data info template"=w174, "Cluster"=w180) -> ("error out"=w184:errorcluster, "source"=w189:T10, "chan.in.files"=w147:i16[])  [unwired: 3 in, 3 out]
            "source" <- w189
            "chan.in.files" <- w147
            n106 = Unbundle By Name(w189) -> ("data path"=w162:string[], "data"=w173:waveform(dbl)[])
            n107 = Index Array(array=w147) -> (element=w146:i16)  [unwired: 1 in]
            n108 = control-ref of="show\nplots"() -> (w164:refnum<vi>)
            n109 = property class="DigNum (strict)"(reference=w164) -> ("Value"=w163:i16)  [unwired: 1 in, 2 out]
            n110 = property on="ch#" class="DigNum (strict)"("Maximum"=w146) -> ()  [unwired: 2 in, 2 out]
            n111 = for {
              tunnel: w162 -> [w208] mode=indexing
              tunnel: [w204] -> w170 mode=indexing
              tunnel: w173 -> [w197] mode=indexing
              tunnel: w175 -> [w199]
              tunnel: [w198] -> w148 mode=indexing
              tunnel: [w196] -> w160
              w203 = "\\" ("regular expression")
              n112 = Reverse String(1:w208) -> (0:w207:string)
              n113 = Match Pattern(string=w207, regular expression=w203) -> (before substring=w201:string, after substring=w206:string)  [unwired: 1 in, 2 out]
              n114 = Match Pattern(string=w206, regular expression=w203) -> (before substring=w202:string)  [unwired: 1 in, 3 out]
              n115 = Concatenate Strings(w202, w203, w201) -> (w205:string)
              n116 = Reverse String(1:w205) -> (0:w204:string)
              n117 = Get Waveform Attribute(5:w199, 6:"info" ("name"), 7:w197) -> (1:w198:T1, 3:w196:waveform(dbl))  [unwired: 1 in, 2 out]
            }
            "allinfos" <- w148
            n118 = Index Array(array=w162) -> (element=w191:string)  [unwired: 1 in]
            n119 = Array Size(array=w162) -> (size(s)=w168:i32)
            n120 = control-ref of="total\nplots"() -> (w169:refnum<vi>)
            n121 = String To Path(string=w191) -> (path=w192:path)
            n122 = In Range and Coerce(upper limit=w168, x=w163, lower limit=0) -> (coerced(x)=w185:i32)  [unwired: 1 out]
            n123 = Strip Path(path=w192) -> (stripped path=w178:path)  [unwired: 1 out]
            n124 = property class="DigNum (strict)"(reference=w169, "Value"=w168) -> ()  [unwired: 1 in, 2 out]
            n125 = Initialize Array(T23 {"dataname"=0, "X-shift"=0, "Y-shift"=0.0, "width"=0, "Color"=16860, "visible"=TRUE, "multiplic."=1.0} ("data select 4"), w185) -> (w186:T28)
            n126 = File/Directory Info(path=w178) -> (last mod=w179:timestamp)  [unwired: 1 in, 6 out]
            n127 = for {
              tunnel: w186 -> [w216] mode=indexing
              tunnel: [w217] -> w187 mode=indexing
              i -> [w213]
              n128 = In Range and Coerce(upper limit=i16 20, x=w213, lower limit=i16 0) -> (coerced(x)=w209:i32)  [unwired: 1 out]
              n129 = Increment(x=w213) -> (x+1=w212:i32)
              n130 = Index Array(array=u32[] [0, 128, 16711680, 65280, 255, 15712512, 65535, 16711935, 8388608, 8421376, 32768, 8388736, 32896, 23039, 6160584, 16731648, 37103, 10420323, 7667456, 11828224, 8421504, 8421504, 8421504, 8421504, 8421504, 8421504, 8421504, 8421504, 8421504, 8421504, 8421504, 8421504, 8421504, 8421504, 8421504, 8421504, 8421504, 8421504, 8421504, 8421504, 8421504, 8421504, 8421504, 8421504, 8421504, 8421504, 8421504, 8421504, 8421504, 8421504, 8421504, 8421504, 8421504, 8421504, 8421504, 8421504, 8421504, 8421504, 8421504, 8421504, 8421504, 8421504, 8421504, 8421504, 8421504, 8421504, 8421504, 8421504, 8421504, 8421504, 8421504, 8421504, 8421504, 8421504, 8421504, 8421504, 8421504, 8421504, 8421504, 8421504, 8421504, 8421504, 8421504, 8421504, 8421504, 8421504, 8421504, 8421504, 8421504, 8421504, 8421504, 8421504, 8421504, 8421504, 8421504, 8421504, 8421504, 8421504, 8421504, 8421504] ("Array 3"), index=w209) -> (element=w210:u32)
              n131 = Bundle By Name(cluster=w216, "dataname"=w212, "Color"=w210) -> (w217:T23)
            }
            n132 = Bundle("last mod"=w179, "stripped path"=w178) -> (→"observeddir":T9)  [unwired: 1 in]
            n133 = call-poly <vilib>:"Waveform Duration.vi"("waveform in"=w160) -> ("duration"=w153:dbl, "waveform out"=w159:waveform(dbl))  [unwired: 8 in, 1 out]
            n134 = Unbundle By Name(w159) -> ("dt"=w155:dbl)
            n135 = Multiply(x=w155, y=w156) -> (x*y=w151:dbl)
            n136 = Multiply(x=w153, y=w156) -> (x*y=w150:dbl)
            n137 = property on="start zero, ms" class="DigNum (strict)"("Maximum"=w150, "Minimum"=w151, "OutOfRngActMax"=w149, "OutOfRngActMin"=w149) -> ()  [unwired: 2 in, 2 out]
            n138 = property on="duration of zero,ms" class="DigNum (strict)"("Maximum"=w150, "Minimum"=w151, "OutOfRngActMax"=w149, "OutOfRngActMin"=w149) -> ()  [unwired: 2 in, 2 out]
            n139 = Multiply(x=w151, y=2.0) -> (x*y=w154:dbl)
            n140 = Divide(x=w150, y=2.0) -> (x/y=w152:dbl)
            n141 = flat-sequence {
              tunnel: w187 -> [w194]
              tunnel: w185 -> [w193]
              tunnel: w172 -> [w195]
              frame #0 {
                n142 = property on="inp.control" class="Arr (strict)"("Value"=w194, "Number of Rows"=w193) -> ()  [unwired: 2 in, 2 out]
              }
              frame #1 {
                n143 = property on="dataname" class="Ring (strict)"("Strings []"=w195) -> ()  [unwired: 2 in, 2 out]
              }
            }
            n144 = control-ref of="wind.,\nms"() -> (w171:refnum<vi>)
            n145 = property on="Property Node" class="DigNum (strict)"(reference=w171, "Minimum"=w154, "Maximum"=w152, "OutOfRngActMax"=w149, "OutOfRngActMin"=w149) -> ()  [unwired: 1 in, 2 out]
            n146 = property class="Splitter"(reference=w183, error in=w184, "Position"=60 ("Splitter Position")) -> (reference out=w182:refnum<vi>, error out=w144:errorcluster)
            n147 = Build Array (concatenate)("***", w170) -> (w172:string[])
            n148 = property on="regime" class="Ring (strict)"(error in=w144, "DisabledEnum"=T22."Enabled" ("Disabled")) -> (error out=w166:errorcluster)  [unwired: 1 in, 1 out]
            n149 = invoke on="regime" class="Ring (strict)" method="Reinit To Default"(error in=w166) -> (error out=w165:errorcluster)  [unwired: 2 in, 2 out]
          }
        }
        n150 = control-ref of="chan.in.files"() -> (w133:refnum<vi>)
        n151 = property class="Arr (strict)"(reference=w133) -> ("Value"=w132:i16[])  [unwired: 1 in, 2 out]
      }
      frame #4 {
        n152 = control-ref of="triple probe"() -> (w248:refnum<vi>)
        n153 = control-ref of="data view"() -> (w253:refnum<vi>)
        n154 = control-ref of="cut.filtered"() -> (w252:refnum<vi>)
        n155 = control-ref of="tripleProbeSetting"() -> (w247:refnum<vi>)
        n156 = control-ref of="spctrgrmClaster"() -> (w249:refnum<vi>)
        n157 = control-ref of="preproc.settings"() -> (w250:refnum<vi>)
        n158 = control-ref of="spectr.filt."() -> (w255:refnum<vi>)
        n159 = control-ref of="inpcontrclaster"() -> (w251:refnum<vi>)
        n160 = control-ref of="data cut"() -> (w254:refnum<vi>)
        n161 = case shown="0, Default" "regime" {
          tunnel: w259 -> [w285 _ _ _]
          tunnel: w257 -> [w276 w1073 w1182 w2008]
          tunnel: w255 -> [w275 w1071 w1188 w2003]
          tunnel: w260 -> [w273 _ _ _]
          tunnel: w258 -> [w270 w1041 _ _]
          tunnel: w254 -> [_ w1044 w1187 w1999]
          tunnel: w253 -> [w267 w1042 w1145 w2006]
          tunnel: w252 -> [w266 w1043 w1185 w2007]
          tunnel: w251 -> [w265 w1040 w1184 w2005]
          tunnel: w250 -> [w264 w1039 w1174 w2010]
          tunnel: w249 -> [w263 w1038 w1157 _]
          tunnel: w248 -> [w262 w1032 w1144 w2002]
          tunnel: w247 -> [w261 w1031 w1143 w1971]
          frame 0, Default {
            n162 = flat-sequence {
              tunnel: w270 -> [_]
              tunnel: w273 -> [w300]
              tunnel: w275 -> [w299]
              tunnel: w276 -> [w296]
              tunnel: w285 -> [w301]
              tunnel: [w301] -> w269
              tunnel: [w300] -> w268
              tunnel: w267 -> [w298]
              tunnel: w266 -> [w297]
              tunnel: w265 -> [w294]
              tunnel: w264 -> [w291]
              tunnel: w263 -> [w290]
              tunnel: w262 -> [w288]
              tunnel: w261 -> [w287]
              tunnel: [w315] -> w274
              tunnel: w269 -> [w315]
              tunnel: w268 -> [w311]
              tunnel: [w376] -> w284
              tunnel: [w373] -> w282
              tunnel: [w374] -> w280
              tunnel: w274 -> [w376]
              tunnel: w284 -> [w386]
              tunnel: [w386] -> w283
              tunnel: w282 -> [w385]
              tunnel: [w385] -> w281
              tunnel: w280 -> [w384]
              tunnel: [w384] -> w279
              tunnel: w283 -> [_]
              tunnel: w281 -> [w447]
              tunnel: w279 -> [w446]
              tunnel: [w439] -> w277
              tunnel: [w427] -> w271
              tunnel: [w837] -> w278
              tunnel: w277 -> [w837]
              tunnel: [w836] -> w272
              tunnel: w271 -> [w836]
              tunnel: w278 -> [w907]
              tunnel: w272 -> [w904]
              frame #0 {
                w286 = FALSE ("Visible")
                w293 = TRUE ("Visible")
                w289 = FALSE ("Visible")
                n163 = property class="Splitter"(reference=w296, "Position"=60 ("Splitter Position")) -> ()  [unwired: 1 in, 2 out]
                n164 = property class="Clust (strict)"(reference=w291, "Visible"=w289) -> ()  [unwired: 1 in, 2 out]
                n165 = property on="Property Node" class="TabCtl (strict)"(reference=w299, "Visible"=w289) -> ()  [unwired: 1 in, 2 out]
                n166 = property class="Clust (strict)"(reference=w290, "Visible"=w289) -> ()  [unwired: 1 in, 2 out]
                n167 = property class="Clust (strict)"(reference=w287, "Visible"=w286) -> ()  [unwired: 1 in, 2 out]
                n168 = property class="WFGraph (strict)"(reference=w288, "Visible"=w286) -> ()  [unwired: 1 in, 2 out]
                n169 = property class="WFGraph (strict)"(reference=w297, "Visible"=w286) -> ()  [unwired: 1 in, 2 out]
                n170 = property class="Clust (strict)"(reference=w294, "Visible"=w293) -> ()  [unwired: 1 in, 2 out]
                n171 = property on="Property Node" class="WFGraph (strict)"(reference=w298, "Visible"=w293) -> (reference out=w292:refnum<vi>)  [unwired: 1 in, 1 out]
                n172 = invoke class="WFGraph (strict)" method="FitControlToPane"(reference=w292) -> ()  [unwired: 2 in, 3 out]
              }
              frame #1 {
                n173 = control-ref of="showwhat"() -> (w305:refnum<vi>)
                n174 = property class="Clust (strict)"(reference=w305) -> ("Value"=w304:T29)  [unwired: 1 in, 2 out]
                n175 = Unbundle By Name(w304) -> ("show one/all"=w303:bool, "ch#"=w302:i32)
                n176 = control-ref of="inp.control"() -> (w314:refnum<vi>)
                n177 = case shown="True" "cleararray" {
                  tunnel: w314 -> [_ w368]
                  tunnel: [FALSE TRUE] -> w310
                  frame False {
                  }
                  frame True {
                    n178 = property class="Arr (strict)"(reference=w368) -> (reference out=w365:refnum<vi>, "Value"=w364:T30)  [unwired: 1 in, 1 out]
                    n179 = for {
                      tunnel: w364 -> [w372] mode=indexing
                      tunnel: [w370] -> w366 mode=indexing
                      tunnel: u16 0 ("dataname") -> [w369]
                      n180 = Bundle By Name(cluster=w372, "dataname"=w369, "visible"=FALSE) -> (w370:T31)
                    }
                    n181 = property class="Arr (strict)"(reference=w365, "Value"=w366) -> ()  [unwired: 1 in, 2 out]
                  }
                }
                n182 = case shown="True" "show all" {
                  tunnel: w314 -> [_ w321]
                  tunnel: w311 -> [_ w320]
                  tunnel: [FALSE TRUE] -> w309
                  tunnel: w303 -> [_ w318]
                  tunnel: w302 -> [_ w317]
                  frame False {
                  }
                  frame True {
                    n183 = case shown="True" w318 {
                      tunnel: w321 -> [w322 w341]
                      tunnel: w320 -> [_ w338]
                      tunnel: w317 -> [_ w336]
                      frame False {
                        n184 = property on="Property Node" class="Arr (strict)"(reference=w322) -> (reference out=w325:refnum<vi>, "Value"=w324:T30)  [unwired: 1 in, 1 out]
                        n185 = for {
                          tunnel: [w330] -> w323 mode=indexing
                          tunnel: w324 -> [w329] mode=indexing
                          i -> [w327]
                          n186 = Increment(x=w327) -> (x+1=w326:i32)
                          n187 = Bundle By Name(cluster=w329, "dataname"=w326, "visible"=TRUE) -> (w330:T31)
                        }
                        n188 = property on="Property Node" class="Arr (strict)"(reference=w325, "Value"=w323) -> ()  [unwired: 1 in, 2 out]
                      }
                      frame True {
                        w340 = 0
                        n189 = property on="Property Node" class="Arr (strict)"(reference=w341) -> (reference out=w342:refnum<vi>, "Value"=w332:T30)  [unwired: 1 in, 1 out]
                        n190 = Array Size(array=w338) -> (size(s)=w337:i32)
                        n191 = for {
                          tunnel: w332 -> [w346] mode=indexing
                          tunnel: [w344] -> w331 mode=indexing
                          tunnel: u16 0 ("dataname") -> [w343]
                          n192 = Bundle By Name(cluster=w346, "dataname"=w343, "visible"=FALSE) -> (w344:T31)
                        }
                        n193 = for {
                          N: w337 -> [_]
                          tunnel: [w361] -> w335 mode=indexing
                          tunnel: w331 -> [w348]
                          tunnel: w338 -> [w358]
                          tunnel: w336 -> [w359]
                          shift-right: [w349] -> _
                          shift-left: w340 -> [w353]
                          shift-right: [w351] -> _
                          shift-left: w340 -> [w352]
                          i -> [w349]
                          n194 = Index Array(array=w358, index=w353) -> (element=w357:i16)
                          n195 = Add(x=w357, y=w352) -> (x+y=w354:i32)
                          n196 = Equal To 0?(x=w349) -> (x = 0?=w356:bool)
                          n197 = Select(t=0, s=w356, f=w354) -> (s? t:f=w351:i32)
                          n198 = Add(x=w351, y=w359) -> (x+y=w350:i32)
                          n199 = Index Array(array=w348, index=w349) -> (element=w347:T31)
                          n200 = Bundle By Name(cluster=w347, "dataname"=w350, "visible"=TRUE) -> (w361:T31)
                        }
                        n201 = Replace Array Subset(array=w331, new element=w335, index=0) -> (w334:T30)
                        n202 = property on="Property Node" class="Arr (strict)"(reference=w342, "Value"=w334) -> ()  [unwired: 1 in, 2 out]
                      }
                    }
                  }
                }
                n203 = control-ref of="return pressed?"() -> (w308:refnum<vi>)
                n204 = property class="Bool (strict)"(reference=w308) -> ("Value"=w306:bool)  [unwired: 1 in, 2 out]
                n205 = Compound Arithmetic op=OR(w310, w309, w306) -> (→"recalculate?":bool)
              }
              frame #2 {
                n206 = local read "source"() -> (w375:T10)
                n207 = Unbundle By Name(w375) -> ("data path"=w374:string[], "data"=w373:waveform(dbl)[])
              }
              frame #3 {
                n208 = Unbundle By Name("param.table") -> ("press after parram.input"=w379:bool, "data info manual input"=w377:string[][])
                n209 = control-ref of="data view"() -> (w378:refnum<vi>)
                n210 = feedback #1() -> (w381:path)  [unwired: 1 in]
                n211 = case shown="True" w379 {
                  selector: w379 -> [_ w392]
                  tunnel: w377 -> [_ w388]
                  tunnel: w381 -> [_ w390]
                  tunnel: w378 -> [_ w391]
                  frame False {
                  }
                  frame True {
                    n212 = Not(x=w392) -> (.not. x?=w395:bool)
                    n213 = call <vilib>:"Check if File or Folder Exists.vi"("path"=w390) -> ("file or folder exists?"=w389:bool)  [unwired: 8 in, 2 out]
                    n214 = property on="param.table" class="Clust"("Visible"=w395) -> (error out=w394:errorcluster)  [unwired: 2 in, 1 out]
                    n215 = case shown="False" w389 {
                      tunnel: w388 -> [w397 w399]
                      tunnel: [w396 w399] -> w387
                      frame False {
                        n216 = property on="data info manual input" class="Tbl (strict)"() -> ("Column Headers[]"=w398:string[])  [unwired: 2 in, 2 out]
                        n217 = Build Array (concatenate)(w398, w397) -> (w396:string[][])
                      }
                      frame True {
                      }
                    }
                    n218 = property on="Property Node" class="WFGraph (strict)"(reference=w391, error in=w394, "Visible"=w392) -> (error out=w393:errorcluster)  [unwired: 1 out]
                    n219 = invoke on="data view" class="WFGraph (strict)" method="FitControlToPane"(error in=w393) -> ()  [unwired: 2 in, 3 out]
                    n220 = call-poly <vilib>:"Write To Spreadsheet File.vi"("2D data"=w387, "file path (dialog if empty)"=w390) -> ()  [unwired: 6 in, 1 out]
                  }
                }
                n221 = case shown="True" "setInfo" {
                  selector: "setInfo" -> [_ w404]
                  tunnel: w384 -> [_ w416]
                  tunnel: [w400 w415] -> w382
                  tunnel: w378 -> [_ w403]
                  tunnel: w381 -> [w400 _]
                  frame False {
                  }
                  frame True {
                    n222 = Index Array(array=w416) -> (element=w405:string)  [unwired: 1 in]
                    n223 = Not(x=w404) -> (.not. x?=w414:bool)
                    n224 = property on="Property Node" class="WFGraph (strict)"(reference=w403, "Visible"=w414) -> (error out=w402:errorcluster)  [unwired: 1 in, 1 out]
                    n225 = String To Path(string=w405) -> (path=w413:path)
                    n226 = property on="param.table" class="Clust"(error in=w402, "Visible"=w404) -> (error out=w401:errorcluster)  [unwired: 1 in, 1 out]
                    n227 = Strip Path(path=w413) -> (stripped path=w408:path)  [unwired: 1 out]
                    n228 = Strip Path(path=w408) -> (name=w409:string)  [unwired: 1 out]
                    n229 = invoke on="param.table" class="Clust" method="FitControlToPane"(error in=w401) -> ()  [unwired: 2 in, 3 out]
                    n230 = Concatenate Strings(w409, ".info.txt" ("string")) -> (w411:string)
                    n231 = Build Path(base path=w408, name or relative path=w411) -> (appended path=w410:path)
                    n232 = call <vilib>:"Check if File or Folder Exists.vi"("path"=w410) -> ("file or folder exists?"=w406:bool, "dup path"=w407:path)  [unwired: 8 in, 1 out]
                    n233 = case shown="False" w406 {
                      tunnel: w407 -> [w417 w420]
                      tunnel: [w417 w419] -> w415
                      frame False {
                      }
                      frame True {
                        n234 = call-poly <vilib>:"Read From Spreadsheet File.vi"("file path (dialog if empty)"=w420) -> ("all rows"=w418:string[][], "new file path (Not A Path if cancelled)"=w419:path)  [unwired: 6 in, 3 out]
                        n235 = property on="data info manual input" class="Tbl (strict)"("Value"=w418) -> ()  [unwired: 2 in, 2 out]
                      }
                    }
                  }
                }
                n236 = feedback-in #1(w382) -> ()
              }
              frame #4 {
                n237 = control-ref of="recalculate?"() -> (w442:refnum<vi>)
                n238 = control-ref of="nextfile"() -> (w426:refnum<vi>)
                n239 = control-ref of="data view"() -> (w423:refnum<vi>)
                n240 = property on="smooth" class="Ring (strict)"("DecKeyBind"=T24 {"Focus"=FALSE, "Control"=FALSE, "Shift"=FALSE, "Key"="<PageDown>"} ("Increment Key Binding"), "IncKeyBind"=T24 {"Focus"=FALSE, "Control"=FALSE, "Shift"=FALSE, "Key"="<PageUp>"} ("Decrement Key Binding")) -> ()  [unwired: 2 in, 2 out]
                n241 = property class="Bool (strict)"(reference=w442) -> ("Value"=w428:bool)  [unwired: 1 in, 2 out]
                n242 = property class="Bool (strict)"(reference=w426) -> ("Value"=w425:bool)  [unwired: 1 in, 2 out]
                n243 = control-ref of="smooth"() -> (w438:refnum<vi>)
                n244 = property class="WFGraph (strict)"(reference=w423) -> ("Value"=w445:waveform(dbl)[])  [unwired: 1 in, 2 out]
                n245 = property class="Ring (strict)"(reference=w438) -> ("Value"=w437:u16)  [unwired: 1 in, 2 out]
                n246 = Or(x=w428, y=w425) -> (x .or. y?=w427:bool)
                n247 = case shown="True" "writedat" {
                  tunnel: w423 -> [_ w458]
                  frame False {
                  }
                  frame True {
                    n248 = Get Date/Time In Seconds() -> (seconds since 1Jan1904=w460:timestamp)
                    n249 = Format Date/Time String(time format string (%c)="%y.%m.%d_%H.%M.%S%2u", seconds (now)=w460) -> (date/time string=w450:string)  [unwired: 1 in]
                    n250 = Concatenate Strings(w450, ".txt" ("string")) -> (w451:string)
                    n251 = Concatenate Strings(w450, ".png" ("string")) -> (w456:string)
                    n252 = flat-sequence {
                      tunnel: w456 -> [w465]
                      tunnel: [w466] -> w459
                      tunnel: [w464] -> w454
                      tunnel: w451 -> [w463]
                      tunnel: [w462] -> w448
                      tunnel: w459 -> [w476]
                      tunnel: w458 -> [w479]
                      tunnel: [w477] -> w455
                      tunnel: w454 -> [w475]
                      tunnel: [w475] -> w453
                      tunnel: [w473] -> w449
                      tunnel: w448 -> [w473]
                      tunnel: w455 -> [w489]
                      tunnel: w453 -> [w482]
                      tunnel: w449 -> [w481]
                      frame #0 {
                        n253 = call <vilib>:"Check if File or Folder Exists.vi"("path"=path "d:/ADCtmp" ("Path")) -> ("file or folder exists?"=w468:bool, "dup path"=w467:path)  [unwired: 8 in, 1 out]
                        n254 = case shown="False" w468 {
                          tunnel: [w470 w472] -> w462
                          tunnel: w467 -> [w471 w472]
                          frame False {
                            n255 = Create Folder(path (use dialog)=w471) -> (created path=w470:path)  [unwired: 2 in, 2 out]
                          }
                          frame True {
                          }
                        }
                        n256 = Build Path(base path=w462, name or relative path=w463) -> (appended path=w464:path)
                        n257 = Build Path(base path=w462, name or relative path=w465) -> (appended path=w466:path)
                      }
                      frame #1 {
                        n258 = invoke class="WFGraph (strict)" method="Get Image"(reference=w479, "image depth"=24 ("Image Depth")) -> (reference out=w477:refnum<vi>, "image data"=w480:T32)  [unwired: 4 in, 4 out]
                        n259 = call <vilib>:"Write PNG File.vi"("compression (default)"=-1, "image data"=w480, "path to PNG file"=w476) -> ()  [unwired: 7 in, 2 out]
                      }
                      frame #2 {
                        n260 = property class="WFGraph (strict)"(reference=w489) -> (reference out=w488:refnum<vi>, "Value"=w487:waveform(dbl)[])  [unwired: 1 in, 1 out]
                        n261 = for {
                          tunnel: w488 -> [w527]
                          tunnel: w487 -> [w505] mode=indexing
                          tunnel: [w514] -> w486 mode=concatenating
                          tunnel: w481 -> [w500]
                          i -> [w513]
                          w517 = 0 ("index")
                          n262 = property class="WFGraph (strict)"(reference=w527, "Active Plot"=w513) -> ("Plot.Plot Name"=w497:string)  [unwired: 1 in, 2 out]
                          n263 = call-poly <vilib>:"Get Waveform Time Array.vi"("waveform in"=w505) -> ("X array"=w526:timestamp[])  [unwired: 9 in, 1 out]
                          n264 = property on="data info template" class="Clust (strict)"() -> (error out=w504:errorcluster, "Value"=w503:T1)  [unwired: 2 in, 1 out]
                          n265 = To Double Precision Float(number=w526) -> (double precision float=w522:dbl[])
                          n266 = Unbundle By Name(w505) -> ("Y"=w518:dbl[])
                          n267 = Concatenate Strings("time_" ("element"), w497) -> (w521:string)
                          n268 = Number To Fractional String(use system decimal point (T)=FALSE, number=w522, precision (6)=i16 7) -> (F-format string=w508:string[])  [unwired: 1 in]
                          n269 = Number To Fractional String(use system decimal point (T)=FALSE, number=w518, precision (6)=i16 7) -> (F-format string=w507:string[])  [unwired: 1 in]
                          n270 = Get Waveform Attribute(4:w504, 5:w503, 6:"info" ("name"), 7:w505) -> (1:w502:T1)  [unwired: 3 out]
                          n271 = Insert Into Array(array=w508, index=w517, new element=w521) -> (w516:string[])
                          n272 = Insert Into Array(array=w507, index=w517, new element=w497) -> (w515:string[])
                          n273 = Build Array(w508, w507) -> (w509:string[][])
                          n274 = Unbundle By Name(w502) -> ("data path"=w494:string, "LastModified"=w495:string)
                          n275 = Build Array(w516, w515) -> (w514:string[][])
                          n276 = Transpose 2D Array(2D array=w509) -> (transposed array=w510:string[][])
                          n277 = Reverse String(1:w494) -> (0:w493:string)
                          n278 = Match Pattern(string=w493, regular expression="\\") -> (before substring=w492:string)  [unwired: 1 in, 3 out]
                          n279 = Reverse String(1:w492) -> (0:w491:string)
                          n280 = Concatenate Strings(w491, "_", w495, ".txt" ("string")) -> (w490:string)
                          n281 = Build Path(base path=w500, name or relative path=w490) -> (appended path=w498:path)
                          n282 = call-poly <vilib>:"Write To Spreadsheet File.vi"("delimiter (\\t)"=",\t" ("delimiter (\\t)"), "format (%s)"="%s", "2D data"=w510, "file path (dialog if empty)"=w498) -> ()  [unwired: 4 in, 1 out]
                        }
                        n283 = Transpose 2D Array(2D array=w486) -> (transposed array=w483:string[][])
                        n284 = call-poly <vilib>:"Write To Spreadsheet File.vi"("delimiter (\\t)"=",\t" ("delimiter (\\t)"), "format (%s)"="%s", "2D data"=w483, "file path (dialog if empty)"=w482) -> ()  [unwired: 4 in, 1 out]
                      }
                    }
                  }
                }
                n285 = property on="AxisX" class="Ring (strict)"() -> ("Value"=w422:u16)  [unwired: 2 in, 2 out]
                n286 = case shown="True" w427 {
                  tunnel: w447 -> [_ w545]
                  tunnel: w446 -> [_ w577]
                  tunnel: [w538 w568] -> w439
                  tunnel: w437 -> [_ w573]
                  tunnel: "wind.,\nms" -> [_ w572]
                  tunnel: "polyn.\norder" -> [_ w571]
                  tunnel: w445 -> [w538 _]
                  tunnel: "aver.\ncolor" -> [_ w559]
                  tunnel: "width" -> [_ w558]
                  tunnel: "show legend" -> [_ w557]
                  tunnel: "path-name" -> [_ w560]
                  tunnel: "smooth" -> [_ w546]
                  tunnel: w423 -> [_ w562]
                  tunnel: w422 -> [_ w551]
                  frame False {
                  }
                  frame True {
                    n287 = Bundle("show legend"=w557, "path-name"=w560, "aver.\ncolor"=w559, "width"=w558) -> (w556:T33)  [unwired: 1 in]
                    n288 = property on="inpcontrclaster" class="Clust (strict)"() -> ("Value"=w543:T6)  [unwired: 2 in, 2 out]
                    n289 = Unbundle By Name(w543) -> ("decimate"=w542:bool, "factor"=w540:i32, "average"=w541:bool)
                    n290 = case shown="True" w542 {
                      tunnel: w545 -> [w578 w582]
                      tunnel: [w578 w579] -> w544
                      tunnel: w541 -> [_ w581]
                      tunnel: w540 -> [_ w580]
                      frame False {
                      }
                      frame True {
                        n291 = for {
                          tunnel: w582 -> [w588] mode=indexing
                          tunnel: w581 -> [w586]
                          tunnel: w580 -> [w583]
                          tunnel: [w584] -> w579 mode=indexing
                          n292 = call-poly <vilib>:"Decimate (single shot).vi"("averaging"=w586, "decimating factor"=w583, "X"=w588) -> ("Decimated Array"=w587:dbl[])  [unwired: 7 in, 1 out]
                          n293 = Bundle By Name(cluster=w588, "Y"=w587) -> (w585:waveform(dbl))
                          n294 = call-poly <vilib>:"Scale Delta t.vi"("scale factor"=w583, "waveform in"=w585) -> ("waveform out"=w584:waveform(dbl))  [unwired: 8 in, 1 out]
                        }
                      }
                    }
                    n295 = case shown="0, Default" w546 {
                      tunnel: w544 -> [w607 w615 w623]
                      tunnel: [0 w610 w618] -> w563
                      tunnel: w562 -> [w602 w609 w617]
                      tunnel: [w601 w608 w616] -> w561
                      frame 0, Default {
                        n296 = Array Size(array=w607) -> (size(s)=w606:i32)
                        n297 = Initialize Array(waveform(dbl) {"t0"=timestamp(0 s since 1904-01-01), "dt"=1.0, "Y"=[]} ("Waveform"), w606) -> (w604:waveform(dbl)[])
                        n298 = property class="WFGraph (strict)"(reference=w602, "Value"=w604) -> (reference out=w601:refnum<vi>)  [unwired: 1 in, 1 out]
                      }
                      frame 1 {
                        n299 = Array Size(array=w615) -> (size(s)=w610:i32)
                        n300 = Multiply(x=2, y=w610) -> (x*y=w611:i32)
                        n301 = Initialize Array(waveform(dbl) {"t0"=timestamp(0 s since 1904-01-01), "dt"=1.0, "Y"=[]} ("Waveform"), w611) -> (w613:waveform(dbl)[])
                        n302 = property class="WFGraph (strict)"(reference=w609, "Value"=w613) -> (reference out=w608:refnum<vi>)  [unwired: 1 in, 1 out]
                      }
                      frame 5 {
                        n303 = Array Size(array=w623) -> (size(s)=w618:i32)
                        n304 = Multiply(x=2, y=w618) -> (x*y=w619:i32)
                        n305 = Initialize Array(waveform(dbl) {"t0"=timestamp(0 s since 1904-01-01), "dt"=1.0, "Y"=[]} ("Waveform"), w619) -> (w621:waveform(dbl)[])
                        n306 = property class="WFGraph (strict)"(reference=w617, "Value"=w621) -> (reference out=w616:refnum<vi>)  [unwired: 1 in, 1 out]
                      }
                    }
                    n307 = control-ref of="inp.control"() -> (w555:refnum<vi>)
                    n308 = control-ref of="allinfos"() -> (w539:refnum<vi>)
                    n309 = property class="Arr (strict)"(reference=w555) -> ("Value"=w554:T30)  [unwired: 1 in, 2 out]
                    n310 = property class="Arr (strict)"(reference=w539) -> ("Value"=w567:T2)  [unwired: 1 in, 2 out]
                    n311 = control-ref of="data info template"() -> (w574:refnum<vi>)
                    n312 = call "plot_selector6.vi"("smooth"=w546, "drawshift"=w563, "allinfos"=w567, "legent-plot"=w556, "inp.control"=w554, "data view"=w561) -> ("data#inp.control#"=w566:cluster{"data #":i32[], "inp.control#":i32[]})
                    n313 = property class="Clust (strict)"(reference=w574) -> ("Value"=w575:T1)  [unwired: 1 in, 2 out]
                    n314 = Unbundle By Name(w566) -> ("data #"=w565:i32[], "inp.control#"=w564:i32[])
                    n315 = for {
                      N -> [w657]
                      tunnel: w565 -> [w692] mode=indexing
                      tunnel: w544 -> [w693]
                      tunnel: w577 -> [w694]
                      tunnel: [w663] -> w568 mode=indexing
                      tunnel: w564 -> [w691] mode=indexing
                      tunnel: w575 -> [w690]
                      tunnel: w574 -> [w662]
                      tunnel: w573 -> [w658]
                      tunnel: w572 -> [w651]
                      tunnel: w571 -> [w689]
                      tunnel: "applyInfo" -> [w661]
                      tunnel: [w659] -> w569 mode=indexing
                      tunnel: [w645] -> w552
                      tunnel: [w657] -> w553
                      i -> [w655]
                      w634 = 1000.0 ("y")
                      w685 = "info" ("name")
                      n316 = Decrement(x=w692) -> (x-1=w670:i32)
                      n317 = Index Array(array=w693, index=w670) -> (element=w688:waveform(dbl))
                      n318 = Index Array(array=w694, index=w670) -> (element=w687:string)
                      n319 = call "InfoRead4.vi"("data info template"=w662, "source path"=w687) -> ("data from *.info.txt"=w666:T34)  [unwired: 3 in]
                      n320 = Get Waveform Attribute(5:w690, 6:w685, 7:w688) -> (1:w684:T1, 3:w686:waveform(dbl))  [unwired: 1 in, 2 out]
                      n321 = Unbundle By Name("zero drift control") -> ("start zero, ms"=w638:dbl, "duration of zero,ms"=w637:dbl, "'0',\nms"=w636:bool)
                      n322 = Bundle By Name(cluster=w684, "data info"=w666) -> (w665:T1)
                      n323 = Set Waveform Attribute(5:w665, 6:w685, 7:w686) -> (3:w669:waveform(dbl))  [unwired: 1 in, 2 out]
                      n324 = Divide(x=w638, y=w634) -> (x/y=w635:dbl)
                      n325 = Divide(x=w637, y=w634) -> (x/y=w640:dbl)
                      n326 = case shown="True" w636 {
                        tunnel: w669 -> [w771 w775]
                        tunnel: [w771 w774] -> w668
                        tunnel: w635 -> [_ w777]
                        tunnel: w640 -> [_ w776]
                        frame False {
                        }
                        frame True {
                          w772 = u16 1 items=["Samples", "Relative Time"] ("start/duration format")
                          n327 = call-poly <vilib>:"Get Waveform Subset.vi"("start/duration format"=w772, "duration"=w776, "start samples/time"=w777, "waveform in"=w775) -> ("waveform out"=w778:waveform(dbl))  [unwired: 2 in, 3 out]
                          n328 = Unbundle By Name(w778) -> ("Y"=w779:dbl[])
                          n329 = call-poly <vilib>:"Mean.vi"("X"=w779) -> ("mean"=w773:dbl)  [unwired: 1 out]
                          n330 = Subtract(x=w775, y=w773) -> (x-y=w774:waveform(dbl))
                        }
                      }
                      n331 = control-ref of="inp.control"() -> (w673:refnum<vi>)
                      n332 = property class="Arr (strict)"(reference=w673) -> ("Value"=w674:T30)  [unwired: 1 in, 2 out]
                      n333 = property on="Y shift" class="DigNum (strict)"() -> ("Value"=w656:dbl)  [unwired: 2 in, 2 out]
                      n334 = Index Array(array=w674, index=w691) -> (element=w672:T31)
                      n335 = Unbundle By Name(w672) -> ("X-shift, ms"=w632:dbl, "Y-shift"=w653:dbl, "multiplic."=w671:dbl)
                      n336 = Multiply(x=w656, y=w655) -> (x*y=w654:dbl)
                      n337 = property on="X shift,ms" class="DigNum (strict)"() -> ("Value"=w633:dbl)  [unwired: 2 in, 2 out]
                      n338 = Add(x=w653, y=w654) -> (x+y=w652:dbl)
                      n339 = Add(x=w633, y=w632) -> (x+y=w631:dbl)
                      n340 = Equal To 0?(x=w631) -> (x = 0?=w683:bool)
                      n341 = Greater Than 0?(x=w631) -> (x > 0?=w679:bool)
                      n342 = Absolute Value(x=w631) -> (abs(x)=w676:dbl)
                      n343 = Add(x=w668, y=w652) -> (x+y=w675:waveform(dbl))
                      n344 = Select(t=1, s=w679, f=2) -> (s? t:f=w680:i32)
                      n345 = Multiply(x=w675, y=w671) -> (x*y=w667:waveform(dbl))
                      n346 = Select(t=0, s=w683, f=w680) -> (s? t:f=w681:i32)
                      n347 = case shown="2" w681 {
                        tunnel: [w780 w794 w802] -> w650
                        tunnel: w676 -> [_ w785 w797]
                        tunnel: w667 -> [w780 w791 w799]
                        frame 0, Default {
                        }
                        frame 1 {
                          n348 = Divide(x=w785, y=1000.0) -> (x/y=w784:dbl)
                          n349 = Unbundle By Name(w791) -> ("Y"=w793:dbl[], "dt"=w783:dbl)
                          n350 = Divide(x=w784, y=w783) -> (x/y=w782:dbl)
                          n351 = To Long Integer(number=w782) -> (32bit integer=w781:i32)
                          n352 = Initialize Array(0.0 ("element"), w781) -> (w790:dbl[])
                          n353 = Insert Into Array(array=w793, index=0, new element=w790) -> (w789:dbl[])
                          n354 = Delete From Array(array=w789, length=w781) -> (array with subset deleted=w792:dbl[])  [unwired: 1 in, 1 out]
                          n355 = Bundle By Name(cluster=w791, "Y"=w792) -> (w794:waveform(dbl))
                        }
                        frame 2 {
                          n356 = Divide(x=w797, y=1000.0) -> (x/y=w800:dbl)
                          n357 = Unbundle By Name(w799) -> ("Y"=w803:dbl[], "dt"=w795:dbl)
                          n358 = Divide(x=w800, y=w795) -> (x/y=w798:dbl)
                          n359 = To Long Integer(number=w798) -> (32bit integer=w796:i32)
                          n360 = Initialize Array(0.0 ("element"), w796) -> (w807:dbl[])
                          n361 = Insert Into Array(array=w803, new element=w807) -> (w806:dbl[])  [unwired: 1 in]
                          n362 = Delete From Array(array=w806, length=w796, index=0) -> (array with subset deleted=w808:dbl[])  [unwired: 1 out]
                          n363 = Bundle By Name(cluster=w799, "Y"=w808) -> (w802:waveform(dbl))
                        }
                      }
                      n364 = Divide(x=w651, y=1000.0) -> (x/y=w644:dbl)
                      n365 = Unbundle By Name(w650) -> ("dt"=w649:dbl)
                      n366 = Divide(x=w644, y=2.0) -> (x/y=w643:dbl)
                      n367 = Divide(x=w643, y=w649) -> (x/y=w647:dbl)
                      n368 = To Long Integer(number=w647) -> (32bit integer=w646:i32)
                      n369 = control-ref of="wind.,\nms"() -> (w641:refnum<vi>)
                      n370 = case shown="1" w658 {
                        tunnel: w650 -> [w703 w707 w723 w740 w755 w759 w766]
                        tunnel: [w703 w707 w724 w738 w754 w759 w764] -> w664
                        tunnel: w665 -> [_ _ _ _ _ _ _]
                        tunnel: w646 -> [_ w709 w722 w742 w753 w761 w768]
                        tunnel: w689 -> [_ w708 w725 w741 _ _ _]
                        tunnel: [_ w706 _ _ _ w760 _] -> w660
                        tunnel: [0 1 0 0 _ 1 0] -> w645
                        tunnel: w641 -> [_ w704 w720 w736 _ _ _]
                        frame 0, Default {
                        }
                        frame 1 {
                          n371 = call-poly <vilib>:"Savitzky-Golay Filter.vi"("polynomial order"=w708, "side points"=w709, "X"=w707) -> ("error"=w712:i32, "Filtered X"=w710:dbl[])  [unwired: 7 in]
                          n372 = Bundle By Name(cluster=w707, "Y"=w710) -> (w711:waveform(dbl))
                          n373 = Not Equal To 0?(x=w712) -> (x != 0?=w713:bool)
                          n374 = case shown="True" w713 {
                            tunnel: [w714 w718] -> w706
                            tunnel: w707 -> [_ w718]
                            tunnel: w711 -> [w714 _]
                            tunnel: w704 -> [_ w716]
                            frame False {
                            }
                            frame True {
                              n375 = property on="Property Node" class="DigNum (strict)"(reference=w716) -> (reference out=w715:refnum<vi>, "Minimum"=w717:dbl)  [unwired: 1 in, 1 out]
                              n376 = property on="Property Node" class="DigNum (strict)"(reference=w715, "Value"=w717) -> ()  [unwired: 1 in, 2 out]
                              n377 = property on="polyn.\norder" class="DigNum (strict)"("Value"=1) -> ()  [unwired: 2 in, 2 out]
                            }
                          }
                        }
                        frame 2 {
                          n378 = call-poly <vilib>:"Savitzky-Golay Filter.vi"("polynomial order"=w725, "side points"=w722, "X"=w723) -> ("error"=w728:i32, "Filtered X"=w726:dbl[])  [unwired: 7 in]
                          n379 = Bundle By Name(cluster=w723, "Y"=w726) -> (w727:waveform(dbl))
                          n380 = Not Equal To 0?(x=w728) -> (x != 0?=w729:bool)
                          n381 = case shown="True" w729 {
                            tunnel: [w730 w735] -> w724
                            tunnel: w723 -> [_ w735]
                            tunnel: w727 -> [w730 _]
                            tunnel: w720 -> [_ w733]
                            frame False {
                            }
                            frame True {
                              n382 = property on="Property Node" class="DigNum (strict)"(reference=w733) -> (reference out=w731:refnum<vi>, "Minimum"=w732:dbl)  [unwired: 1 in, 1 out]
                              n383 = property on="Property Node" class="DigNum (strict)"(reference=w731, "Value"=w732) -> ()  [unwired: 1 in, 2 out]
                              n384 = property on="polyn.\norder" class="DigNum (strict)"("Value"=1) -> ()  [unwired: 2 in, 2 out]
                            }
                          }
                        }
                        frame 3 {
                          n385 = call-poly <vilib>:"Savitzky-Golay Filter.vi"("polynomial order"=w741, "side points"=w742, "X"=w740) -> ("error"=w745:i32, "Filtered X"=w743:dbl[])  [unwired: 7 in]
                          n386 = Bundle By Name(cluster=w740, "Y"=w743) -> (w744:waveform(dbl))
                          n387 = Not Equal To 0?(x=w745) -> (x != 0?=w746:bool)
                          n388 = case shown="True" w746 {
                            tunnel: [w747 w751] -> w739
                            tunnel: w740 -> [_ w751]
                            tunnel: w744 -> [w747 _]
                            tunnel: w736 -> [_ w748]
                            frame False {
                            }
                            frame True {
                              n389 = property on="Property Node" class="DigNum (strict)"(reference=w748) -> (reference out=w749:refnum<vi>, "Minimum"=w750:dbl)  [unwired: 1 in, 1 out]
                              n390 = property on="Property Node" class="DigNum (strict)"(reference=w749, "Value"=w750) -> ()  [unwired: 1 in, 2 out]
                              n391 = property on="polyn.\norder" class="DigNum (strict)"("Value"=1) -> ()  [unwired: 2 in, 2 out]
                            }
                          }
                          n392 = Subtract(1:w739, 2:w740) -> (0:w738:waveform(dbl))  [unwired: 1 in, 1 out]
                        }
                        frame 4 {
                          n393 = Unbundle By Name(w755) -> ("Y"=w756:dbl[])
                          n394 = call <vilib>:"Median Filter.vi"("left rank"=w753, "X"=w756) -> ("Filtered X"=w757:dbl[])  [unwired: 8 in, 1 out]
                          n395 = Bundle By Name(cluster=w755, "Y"=w757) -> (w754:waveform(dbl))
                        }
                        frame 5 {
                          n396 = Unbundle By Name(w759) -> ("Y"=w762:dbl[])
                          n397 = call <vilib>:"Median Filter.vi"("left rank"=w761, "X"=w762) -> ("Filtered X"=w763:dbl[])  [unwired: 8 in, 1 out]
                          n398 = Bundle By Name(cluster=w759, "Y"=w763) -> (w760:waveform(dbl))
                        }
                        frame 6 {
                          n399 = Unbundle By Name(w766) -> ("Y"=w769:dbl[])
                          n400 = call <vilib>:"Median Filter.vi"("left rank"=w768, "X"=w769) -> ("Filtered X"=w770:dbl[])  [unwired: 8 in, 1 out]
                          n401 = Bundle By Name(cluster=w766, "Y"=w770) -> (w765:waveform(dbl))
                          n402 = Subtract(1:w765, 2:w766) -> (0:w764:waveform(dbl))  [unwired: 1 in, 1 out]
                        }
                      }
                      n403 = case shown="True" w661 {
                        tunnel: w664 -> [w696 w699]
                        tunnel: [w696 w701] -> w663
                        tunnel: w662 -> [_ w700]
                        tunnel: [w695 w698] -> w659
                        tunnel: w660 -> [w695 w697]
                        frame False {
                        }
                        frame True {
                          n404 = call "Normaliz4.vi"("data info template"=w700, "waveform in"=w699) -> ("waveform out"=w701:waveform(dbl))  [unwired: 3 in]
                          n405 = call "Normaliz4.vi"("data info template"=w700, "waveform in"=w697) -> ("waveform out"=w698:waveform(dbl))  [unwired: 3 in]
                        }
                      }
                    }
                    n406 = control-ref of="data view"() -> (w576:refnum<vi>)
                    n407 = property on="visible\nplots" class="DigNum (strict)"("Value"=w553) -> ()  [unwired: 2 in, 2 out]
                    n408 = case "x-axis scaling" shown="2" w551 {
                      tunnel: w576 -> [w816 w820 w825]
                      tunnel: w568 -> [w815 _ _]
                      tunnel: [w810 w818 w823] -> w547
                      frame 0, Default {
                        # "index"
                        n409 = Index Array(array=w815) -> (element=w814:waveform(dbl))  [unwired: 1 in]
                        n410 = Unbundle By Name(w814) -> ("dt"=w813:dbl)
                        n411 = Reciprocal(x=w813) -> (1/x=w812:dbl)
                        n412 = property on="Property Node" class="WFGraph (strict)"(reference=w816, "XScale.FormatString"="%d" ("X Scale.Format String"), "XScale.Multiplier"=w812, "XScale.NameLbl.Text"="index" ("X Scale.Name Label.Text")) -> (reference out=w810:refnum<vi>)  [unwired: 1 in, 1 out]
                      }
                      frame 1 {
                        # "time, s"
                        n413 = property on="Property Node" class="WFGraph (strict)"(reference=w820, "XScale.FormatString"="%#.7f" ("X Scale.Format String"), "XScale.Multiplier"=1.0 ("X Scale.Offset and Multiplier:Multiplier"), "XScale.NameLbl.Text"="time, s" ("X Scale.Name Label.Text")) -> (reference out=w818:refnum<vi>)  [unwired: 1 in, 1 out]
                      }
                      frame 2 {
                        # "time, ms"
                        n414 = property on="Property Node" class="WFGraph (strict)"(reference=w825, "XScale.FormatString"="%#.7f" ("X Scale.Format String"), "XScale.Multiplier"=1000.0 ("X Scale.Offset and Multiplier:Multiplier"), "XScale.NameLbl.Text"="time, ms" ("X Scale.Name Label.Text")) -> (reference out=w823:refnum<vi>)  [unwired: 1 in, 1 out]
                      }
                    }
                    n415 = case shown="0, Default" w552 {
                      tunnel: w547 -> [w625 w629]
                      tunnel: w568 -> [w624 w627]
                      tunnel: w569 -> [_ w630]
                      frame 0, Default {
                        n416 = property class="WFGraph (strict)"(reference=w625, "Value"=w624) -> ()  [unwired: 1 in, 2 out]
                      }
                      frame 1 {
                        n417 = Insert Into Array(array=w627, index=0, new element=w630) -> (w628:waveform(dbl)[])
                        n418 = property class="WFGraph (strict)"(reference=w629, "Value"=w628) -> ()  [unwired: 1 in, 2 out]
                      }
                    }
                    n419 = property on="Property Node" class="WFGraph (strict)"(reference=w547) -> (reference out=w549:refnum<vi>, "CrsrList"=w550:T27)  [unwired: 1 in, 1 out]
                    n420 = for {
                      tunnel: w550 -> [w600] mode=indexing
                      tunnel: [w590] -> w548 mode=indexing
                      w589 = i16 7 ("precision (6)")
                      n421 = Unbundle By Name(w600) -> ("Position"=w592:cluster{"X":dbl, "Y":dbl})
                      n422 = Unbundle By Name(w592) -> ("X"=w598:dbl, "Y"=w594:dbl)
                      n423 = Number To Fractional String(use system decimal point (T)=FALSE, number=w598, precision (6)=w589) -> (F-format string=w597:string)  [unwired: 1 in]
                      n424 = Number To Fractional String(use system decimal point (T)=FALSE, number=w594, precision (6)=w589) -> (F-format string=w593:string)  [unwired: 1 in]
                      n425 = Concatenate Strings(w597, "\n" ("string"), w593) -> (w591:string)
                      n426 = Bundle By Name(cluster=w600, "Name"=w591) -> (w590:T25)
                    }
                    n427 = property on="Property Node" class="WFGraph (strict)"(reference=w549, "CrsrList"=w548) -> ()  [unwired: 1 in, 2 out]
                  }
                }
                n428 = case shown="6" "smooth" {
                  tunnel: [w528 w529 w530 w531 w533 w535 w537] -> w432
                  tunnel: TRUE -> [_ w529 w530 w531 w533 w535 w537]
                  tunnel: FALSE -> [w528 _ _ _ w532 w534 w536]
                  tunnel: [w528 w529 w530 w531 w532 w534 w536] -> w424
                  frame 0, Default {
                  }
                  frame 1 {
                  }
                  frame 2 {
                  }
                  frame 3 {
                  }
                  frame 4 {
                  }
                  frame 5 {
                  }
                  frame 6 {
                  }
                }
                n429 = property on="width" class="DigNum (strict)"("Visible"=w432) -> ()  [unwired: 2 in, 2 out]
                n430 = property on="wind.,\nms" class="DigNum (strict)"("Visible"=w432) -> ()  [unwired: 2 in, 2 out]
                n431 = property on="aver.\ncolor" class="ColBox"("Visible"=w432) -> ()  [unwired: 2 in, 2 out]
                n432 = property on="polyn.\norder" class="DigNum (strict)"("Visible"=w424) -> ()  [unwired: 2 in, 2 out]
              }
              frame #5 {
                n433 = control-ref of="data view"() -> (w827:refnum<vi>)
                n434 = Or(x="scale fit", y="scalefit2") -> (x .or. y?=w832:bool)
                n435 = case shown="True" w832 {
                  tunnel: w827 -> [_ w899]
                  frame False {
                  }
                  frame True {
                    w900 = u8 1 ("X Scale.Scale Fit")
                    w901 = 0 ("Active X Scale")
                    n436 = property on="Property Node" class="WFGraph (strict)" props=["ActXScl", "ActYScl", "XScale", "ScaleFit", "YScale", "ScaleFit", "Value"](reference=w899, "ActXScl"=w901, "ActYScl"=w901, "XScale.ScaleFit"=w900, "YScale.ScaleFit"=w900) -> ()  [unwired: 1 in, 3 out]
                  }
                }
                n437 = property on="Property Node" class="WFGraph (strict)"(reference=w827, "Cursor.SelColor"=u32 16777225) -> ()  [unwired: 1 in, 2 out]
                n438 = case shown="True" "curs.0" {
                  selector: "curs.0" -> [w838 w843]
                  tunnel: w827 -> [w839 w844]
                  frame False {
                    n439 = property on="Property Node" class="WFGraph (strict)"(reference=w839, "Active Cursor"=u32 0, "Cursor.Visible"=w838) -> (reference out=w842:refnum<vi>)  [unwired: 1 in, 1 out]
                    n440 = property on="Property Node" class="WFGraph (strict)"(reference=w842, "Active Cursor"=1 ("Active Y Scale"), "Cursor.Visible"=w838) -> ()  [unwired: 1 in, 2 out]
                  }
                  frame True {
                    n441 = case shown="False" "curs." {
                      tunnel: w844 -> [w871 w885]
                      tunnel: [w873 _] -> w848
                      tunnel: w843 -> [_ _]
                      frame False {
                        w850 = i16 7 ("precision (6)")
                        w852 = 1 ("Active Y Scale")
                        w863 = u32 0 ("Active Cursor")
                        n442 = property on="Property Node" class="WFGraph (strict)"(reference=w871, "Active Cursor"=w863) -> (reference out=w874:refnum<vi>, "Cursor.Cursor Position"=w878:T35, "Cursor.Cursor Index"=w877:i32)  [unwired: 1 in, 1 out]
                        n443 = property on="Property Node" class="WFGraph (strict)"(reference=w874, "Active Cursor"=w852) -> (reference out=w854:refnum<vi>, "Cursor.Cursor Position"=w876:T35, "Cursor.Cursor Index"=w875:i32)  [unwired: 1 in, 1 out]
                        n444 = Unbundle By Name(w878) -> ("Cursor X"=w865:dbl, "Cursor Y"=w864:dbl)
                        n445 = Unbundle By Name(w876) -> ("Cursor X"=w856:dbl, "Cursor Y"=w855:dbl)
                        n446 = Number To Fractional String(use system decimal point (T)=FALSE, number=w865) -> (F-format string=w869:string)  [unwired: 2 in]
                        n447 = Number To Fractional String(use system decimal point (T)=FALSE, number=w864) -> (F-format string=w866:string)  [unwired: 2 in]
                        n448 = Bundle By Name(cluster=T4 {"X"=0.0, "Y"=0.0, "ind"=0, "X1"=0.0, "Y1"=0.0, "ind1"=0} ("cursors"), "X"=w865, "Y"=w864, "ind"=w877, "X1"=w856, "Y1"=w855, "ind1"=w875) -> (w873:T4)
                        n449 = Number To Fractional String(use system decimal point (T)=FALSE, number=w856, precision (6)=w850) -> (F-format string=w860:string)  [unwired: 1 in]
                        n450 = Number To Fractional String(use system decimal point (T)=FALSE, number=w855, precision (6)=w850) -> (F-format string=w857:string)  [unwired: 1 in]
                        n451 = Concatenate Strings(w869, "\n" ("string"), w866) -> (w862:string)
                        n452 = property on="Property Node" class="WFGraph (strict)"(reference=w854, "Active Cursor"=w863, "Cursor.Cursor Name"=w862) -> (reference out=w853:refnum<vi>)  [unwired: 1 in, 1 out]
                        n453 = Concatenate Strings(w860, "\n" ("string"), w857) -> (w851:string)
                        n454 = property on="Property Node" class="WFGraph (strict)"(reference=w853, "Active Cursor"=w852, "Cursor.Cursor Name"=w851) -> ()  [unwired: 1 in, 2 out]
                      }
                      frame True {
                        w879 = 0 ("Active Y Scale")
                        w893 = 2.0 ("y")
                        n455 = property on="Property Node" class="WFGraph (strict)"(reference=w885, "ActYScl"=w879, "ActXScl"=w879) -> (reference out=w884:refnum<vi>, "XScale.Range"=w898:T36, "YScale.Range"=w897:T36)  [unwired: 1 in, 1 out]
                        n456 = Unbundle By Name "x scale"(w898) -> ("Maximum"=w896:dbl, "Minimum"=w890:dbl)
                        n457 = Unbundle By Name "y scale"(w897) -> ("Maximum"=w895:dbl, "Minimum"=w888:dbl)
                        n458 = Subtract(x=w896, y=w890) -> (x-y=w894:dbl)
                        n459 = Subtract(x=w895, y=w888) -> (x-y=w892:dbl)
                        n460 = Divide(x=w894, y=w893) -> (x/y=w891:dbl)
                        n461 = Divide(x=w892, y=w893) -> (x/y=w889:dbl)
                        n462 = Add(x=w891, y=w890) -> (x+y=w887:dbl)
                        n463 = Add(x=w889, y=w888) -> (x+y=w886:dbl)
                        n464 = Bundle(w887, w886) -> (w882:cluster{dbl, dbl})  [unwired: 1 in]
                        n465 = property on="Property Node" class="WFGraph (strict)"(reference=w884, "Active Cursor"=w879, "Cursor.Cursor Position"=w882) -> (reference out=w881:refnum<vi>)  [unwired: 1 in, 1 out]
                        n466 = property on="Property Node" class="WFGraph (strict)"(reference=w881, "Active Cursor"=1 ("Active Y Scale"), "Cursor.Cursor Position"=w882) -> (reference out=w880:refnum<vi>)  [unwired: 1 in, 1 out]
                        n467 = property on="Property Node" class="WFGraph (strict)"(reference=w880, "ActPaletteTool"=w879) -> ()  [unwired: 1 in, 2 out]
                      }
                    }
                    "cursors" <- w848
                    n468 = property on="Property Node" class="WFGraph (strict)"(reference=w844, "Active Cursor"=u32 0, "Cursor.Visible"=w843) -> (reference out=w847:refnum<vi>)  [unwired: 1 in, 1 out]
                    n469 = property on="Property Node" class="WFGraph (strict)"(reference=w847, "Active Cursor"=1 ("Active Y Scale"), "Cursor.Visible"=w843) -> ()  [unwired: 1 in, 2 out]
                  }
                }
                n470 = property class="WFGraph (strict)"(reference=w827, "Active Cursor"=u32 2, "Cursor.Visible"="\"0\" line", "Cursor.Cursor Color"="0-color") -> ()  [unwired: 1 in, 2 out]
              }
              frame #6 {
                n471 = control-ref of="data cut"() -> (w905:refnum<vi>)
                n472 = property class="Clust (strict)"(reference=w905) -> ("Value"=w903:T11)  [unwired: 1 in, 2 out]
                n473 = control-ref of="data view"() -> (w902:refnum<vi>)
                n474 = case shown="True" w904 {
                  tunnel: w907 -> [_ w920]
                  tunnel: [w908 w919] -> w906
                  tunnel: w903 -> [w908 _]
                  tunnel: w902 -> [_ w917]
                  frame False {
                  }
                  frame True {
                    n475 = property on="Property Node" class="WFGraph (strict)"(reference=w917) -> (reference out=w916:refnum<vi>, "XScale.Range"=w923:T36)  [unwired: 1 in, 1 out]
                    n476 = Unbundle By Name(w923) -> ("Minimum"=w914:dbl, "Maximum"=w913:dbl)
                    n477 = control-ref of="data info template"() -> (w918:refnum<vi>)
                    n478 = property on="AxisX" class="Ring (strict)"() -> ("Value"=w915:u16)  [unwired: 2 in, 2 out]
                    n479 = for {
                      tunnel: w915 -> [w937]
                      tunnel: [w933] -> w922 mode=indexing
                      tunnel: w914 -> [w932]
                      tunnel: w913 -> [w934]
                      tunnel: w920 -> [w930] mode=indexing
                      tunnel: [w936] -> w921 mode=indexing
                      tunnel: [w935] -> w925 mode=indexing
                      tunnel: [w932] -> w924 mode=indexing
                      tunnel: w918 -> [w931]
                      tunnel: w916 -> [w929]
                      tunnel: [w927] -> w912 mode=indexing
                      i -> [w928]
                      n480 = property on="Property Node" class="WFGraph (strict)"(reference=w929, "Active Plot"=w928) -> ("Plot.Plot Name"=w927:string)  [unwired: 1 in, 2 out]
                      n481 = call "cut1.vi"("start/duration format"=w937, "data info template"=w931, "input"=w930, "open interval? (T)"=FALSE, "cut  end"=w934, "cut start"=w932) -> ("Part of input"=w933:waveform(dbl), "short cut data lables"=w935:string, "cut data lables"=w936:string)
                    }
                    n482 = Bundle By Name(cluster=T11 {"data offset array"=[], "data cut array"=[], "data lables"=[], "short data lables"=[]} ("output cluster"), "data cut array"=w922, "data lables"=w921, "short data lables"=w925, "data offset array"=w924) -> (w919:T11)
                    n483 = Insert Into Array(array=w912, index=0, new element="AllPlots" ("new element/subarray")) -> (w910:string[])
                    n484 = property on="picker" class="Ring (strict)"("Strings []"=w910) -> ()  [unwired: 2 in, 2 out]
                  }
                }
                "data cut" <- w906
              }
              frame #7 {
                n485 = property on="listOfProfiles" class="Arr (strict)"() -> ("Value"=w939:path[])  [unwired: 2 in, 2 out]
                n486 = property on="picker" class="Ring (strict)"() -> ("NumItems"=w947:u32)  [unwired: 2 in, 2 out]
                n487 = Equal To 0?(x="picker") -> (x = 0?=w944:bool)
                n488 = control-ref of="data view"() -> (w942:refnum<vi>)
                n489 = case shown="True" w944 {
                  tunnel: [u32 1 w956] -> w946
                  tunnel: w947 -> [_ w957]
                  tunnel: [TRUE FALSE] -> w943
                  frame False {
                  }
                  frame True {
                    n490 = Decrement(x=w957) -> (x-1=w956:u32)
                  }
                }
                n491 = case shown="True" "XY" {
                  tunnel: w939 -> [_ _]
                  frame False {
                  }
                  frame True {
                    n492 = Open VI Reference(vi path=path "subvi/XYQuickView.vi") -> (vi reference=w976:refnum<vi>)  [unwired: 5 in, 1 out]
                    n493 = invoke class="VI" method="Run VI"(reference=w976, "Wait until done"=FALSE ("Wait Until Done")) -> (reference out=w978:refnum<vi>)  [unwired: 3 in, 4 out]
                    n494 = invoke class="VI" method="FP.Open"(reference=w978, "Activate"=TRUE ("Activate?")) -> ()  [unwired: 3 in, 5 out]
                  }
                }
                n495 = control-ref of="dataCutCluster"() -> (w941:refnum<vi>)
                n496 = property on="write" class="Bool"("Visible"=w943) -> ()  [unwired: 2 in, 2 out]
                n497 = property on="AxisX" class="Ring (strict)"() -> ("Value"=w951:u16)  [unwired: 2 in, 2 out]
                n498 = case shown="True" "write" {
                  tunnel: w946 -> [_ w963]
                  tunnel: w944 -> [_ w962]
                  tunnel: "picker" -> [_ w961]
                  tunnel: w942 -> [_ w960]
                  tunnel: w941 -> [_ w959]
                  frame False {
                  }
                  frame True {
                    n499 = for {
                      N: w963 -> [_]
                      tunnel: [w971] -> _
                      tunnel: w962 -> [w970]
                      tunnel: w961 -> [w968]
                      tunnel: w959 -> [w966]
                      tunnel: w960 -> [w965]
                      tunnel: [w964] -> w958
                      i -> [w969]
                      n500 = case shown="False" w970 {
                        tunnel: [w972 w974] -> w967
                        tunnel: w969 -> [_ w974]
                        tunnel: w968 -> [w973 _]
                        frame False {
                          n501 = Decrement(x=w973) -> (x-1=w972:i32)
                        }
                        frame True {
                        }
                      }
                      n502 = call "writeCursors.vi"("plotNumber"=w967, "dataCutCluster"=w966, "WaveformGraph in"=w965) -> (2:"listOfProfiles"=w964:path[], 3:"listOfProfiles"=w971:string[])  [unwired: 7 in]
                    }
                    n503 = property on="listOfProfiles" class="Arr (strict)"("Value"=w958) -> ()  [unwired: 2 in, 2 out]
                  }
                }
                n504 = case shown="True" "points" {
                  tunnel: w942 -> [_ w988]
                  tunnel: w951 -> [_ w987]
                  tunnel: "howmany" -> [_ w986]
                  tunnel: "step, ms" -> [_ w985]
                  tunnel: "picker" -> [_ w984]
                  tunnel: w946 -> [_ w983]
                  tunnel: w944 -> [_ w982]
                  tunnel: w941 -> [_ w981]
                  frame False {
                  }
                  frame True {
                    n505 = for {
                      N: w983 -> [_]
                      tunnel: w988 -> [w998]
                      tunnel: w987 -> [w997]
                      tunnel: w986 -> [w996]
                      tunnel: w985 -> [w995]
                      tunnel: w982 -> [w990]
                      tunnel: w984 -> [w993]
                      tunnel: w981 -> [w991]
                      tunnel: [w989] -> w980
                      i -> [w994]
                      n506 = case shown="True" w990 {
                        tunnel: [w999 w1001] -> w992
                        tunnel: w994 -> [_ w1001]
                        tunnel: w993 -> [w1000 _]
                        frame False {
                          n507 = Decrement(x=w1000) -> (x-1=w999:i32)
                        }
                        frame True {
                        }
                      }
                      n508 = call "createCursors.vi"("xAxisFormat"=w997, "plotNumber"=w992, "howManyPoints"=w996, "step, ms"=w995, "sourceGraph"=w998, "write"=w990, "dataCutCluster"=w991) -> ("listOfProfilesPath"=w989:path[])  [unwired: 4 in]
                    }
                    n509 = property on="listOfProfiles" class="Arr (strict)"("Value"=w980) -> ()  [unwired: 2 in, 2 out]
                  }
                }
              }
              frame #8 {
                n510 = disable-structure shown="Enabled" {
                  frame Disabled {
                    n511 = event shown="[1] \"data view\": Mouse Down" {
                      selector: _ -> [_ _]
                      dyn-events: _ -> [_ _]
                      timeout: 100 -> [_ _]
                      event Timeout {
                        n512 = event-data() -> ()  [unwired: 1 in, 3 out]
                      }
                      event "data view": Mouse Down {
                        n513 = event-data() -> ("Coords"=w1005:T37, "PlatMods"=w1004:T38)  [unwired: 1 in, 6 out]
                        n514 = Unbundle By Name(w1004) -> ("Ctrl"=w1003:bool)
                        n515 = case shown="True" w1003 {
                          tunnel: w1005 -> [_ w1019]
                          frame False {
                          }
                          frame True {
                            w1020 = 0 ("X Scale")
                            n516 = control-ref of="data view"() -> (w1007:refnum<vi>)
                            n517 = invoke on="Invoke Node" class="WFGraph (strict)" method="Map Coords To XY"(reference=w1007, "Coords"=w1019, "X Scale"=w1020, "Y Scale"=w1020) -> (reference out=w1006:refnum<vi>, "XY"=w1010:cluster{"X":dbl, "Y":dbl})  [unwired: 3 in, 5 out]
                            n518 = Bundle By Name(cluster=T25 {"Name"="", "Color"=0, "Style"=0, "Point Style"=0, "Name Visible"=FALSE, "Allow Drag"=FALSE, "Cursor Mode"=0, "Plot"=0, "Index"=0, "Position"={"X"=0.0, "Y"=0.0}, "X Scale"=0, "Y Scale"=0, "Watch Plots"=[], "Watch All Plots"=FALSE, "Plot Area"=0, "Label Offset"={"X"=0.0, "Y"=0.0}} ("element"), "Cursor Mode"=u32 0, "Name Visible"=TRUE ("Watch All Plots"), "Style"=u8 0, "Point Style"=u8 2, "Position"=w1010, "Allow Drag"=TRUE) -> (w1016:T25)
                            n519 = property on="Property Node" class="WFGraph (strict)"(reference=w1006) -> (reference out=w1008:refnum<vi>, "CrsrList"=w1018:T27)  [unwired: 1 in, 1 out]
                            n520 = Build Array (concatenate)(w1018, w1016) -> (w1011:T27)
                            n521 = property on="Property Node" class="WFGraph (strict)"(reference=w1008, "CrsrList"=w1011) -> ()  [unwired: 1 in, 2 out]
                          }
                        }
                      }
                    }
                  }
                  frame Enabled {
                  }
                }
              }
              frame #9 {
                n522 = control-ref of="data view"() -> (w1021:refnum<vi>)
                n523 = case shown="True" "clear" {
                  tunnel: w1021 -> [w1023 w1025]
                  tunnel: [w1023 w1024] -> _
                  frame False {
                  }
                  frame True {
                    n524 = property on="Property Node" class="WFGraph (strict)"(reference=w1025) -> (reference out=w1026:refnum<vi>, "CrsrList"=w1029:T27)  [unwired: 1 in, 1 out]
                    n525 = Array Subset(array=w1029, length=3) -> (w1027:T27)  [unwired: 1 in]
                    n526 = property on="Property Node" class="WFGraph (strict)"(reference=w1026, "CrsrList"=w1027) -> (reference out=w1024:refnum<vi>)  [unwired: 1 in, 1 out]
                  }
                }
              }
            }
          }
          frame 1 {
            w1030 = FALSE ("Visible")
            w1037 = FALSE ("Visible")
            n527 = invoke on="Invoke Node" class="TabCtl (strict)" method="FitControlToPane"(reference=w1071) -> (reference out=w1070:refnum<vi>)  [unwired: 2 in, 2 out]
            n528 = property class="Clust (strict)"(reference=w1044) -> ("Value"=w1060:T11)  [unwired: 1 in, 2 out]
            n529 = property on="Property Node" class="WFGraph (strict)"(reference=w1042, "Visible"=FALSE) -> ()  [unwired: 1 in, 2 out]
            n530 = property class="Splitter"(reference=w1041, "Position"=21 ("Splitter Position")) -> ()  [unwired: 1 in, 2 out]
            n531 = property class="Splitter"(reference=w1073, "Position"=25 ("Position:Top")) -> ()  [unwired: 1 in, 2 out]
            n532 = property on="PSD" class="WFGraph (strict)"() -> ("CrsrList"=w1077:T27)  [unwired: 2 in, 2 out]
            n533 = property on="PSD" class="WFGraph (strict)"("YScale.Mapping Mode"="lin/log") -> ()  [unwired: 2 in, 2 out]
            n534 = property on="Spectrogram" class="IntGraph (strict)"("ZScale.Mapping Mode"="lin/log") -> ()  [unwired: 2 in, 2 out]
            n535 = property on="singletoneresult" class="WFGraph (strict)"("Visible"="show") -> ()  [unwired: 2 in, 2 out]
            n536 = property class="Clust (strict)"(reference=w1031, "Visible"=w1030) -> ()  [unwired: 1 in, 2 out]
            n537 = property class="Clust (strict)"(reference=w1039, "Visible"=w1037) -> ()  [unwired: 1 in, 2 out]
            n538 = property class="WFGraph (strict)"(reference=w1032, "Visible"=w1030) -> ()  [unwired: 1 in, 2 out]
            n539 = property class="Clust (strict)"(reference=w1040, "Visible"=w1037) -> ()  [unwired: 1 in, 2 out]
            n540 = property class="WFGraph (strict)"(reference=w1043, "Visible"=w1037) -> ()  [unwired: 1 in, 2 out]
            n541 = property class="Clust (strict)"(reference=w1038, "Visible"=w1037) -> ()  [unwired: 1 in, 2 out]
            n542 = Unbundle By Name(w1060) -> ("data cut array"=w1061:waveform(dbl)[], "short data lables"=w1036:string[])  [unwired: 2 out]
            n543 = property on="Property Node" class="TabCtl (strict)"(reference=w1070, "Visible"=TRUE) -> ()  [unwired: 1 in, 2 out]
            n544 = Index Array(array=w1077, index=1) -> (element=w1075:T25)
            n545 = Index Array(array=w1077, index=0) -> (element=w1079:T25)
            n546 = property on="channel" class="Ring (strict)"("DecKeyBind"=T24 {"Focus"=FALSE, "Control"=FALSE, "Shift"=FALSE, "Key"="<PageDown>"} ("Decrement Key Binding"), "IncKeyBind"=T24 {"Focus"=FALSE, "Control"=FALSE, "Shift"=FALSE, "Key"="<PageUp>"} ("Increment Key Binding")) -> ()  [unwired: 2 in, 2 out]
            n547 = Unbundle By Name("bandstop") -> ("apply\nfilter"=w1067:bool, "filter structure option"=w1066:T15, "filter type"=w1065:T14, "order"=w1064:i32)
            n548 = Unbundle By Name(w1075) -> ("Position.X"=w1074:dbl)
            n549 = Unbundle By Name(w1079) -> ("Position.X"=w1078:dbl)
            n550 = Array Size(array=w1036) -> (size(s)=w1035:i32)
            n551 = control-ref of="Spectrogram"() -> (w1053:refnum<vi>)
            n552 = control-ref of="return pressed?"() -> (w1063:refnum<vi>)
            n553 = case "bandstop" shown="True" w1067 {
              tunnel: w1074 -> [_ w1130]
              tunnel: w1078 -> [_ w1129]
              tunnel: w1064 -> [_ w1128]
              tunnel: w1065 -> [_ w1127]
              tunnel: w1066 -> [_ w1126]
              tunnel: w1061 -> [_ w1125]
              tunnel: w1060 -> [_ w1124]
              tunnel: w1044 -> [_ w1121]
              frame False {
              }
              frame True {
                n554 = for {
                  tunnel: w1130 -> [w1138]
                  tunnel: w1129 -> [w1137]
                  tunnel: w1128 -> [w1135]
                  tunnel: w1127 -> [w1134]
                  tunnel: w1126 -> [w1133]
                  tunnel: w1125 -> [w1132] mode=indexing
                  tunnel: [w1131] -> w1123 mode=indexing
                  n555 = Unbundle By Name(w1132) -> ("dt"=w1139:dbl)
                  n556 = Reciprocal(x=w1139) -> (1/x=w1136:dbl)
                  n557 = call <vilib>:"Butterworth Coefficients.vi"("filter structure option"=w1133, "order"=w1135, "filter type"=w1134, "low cutoff freq: fl"=w1137, "high cutoff freq: fh"=w1138, "sampling freq: fs"=w1136) -> ("IIR Filter Cluster"=w1141:T39)  [unwired: 4 in, 1 out]
                  n558 = call-poly <vilib>:"Zero Phase Filter.vi"("IIR Filter Cluster"=w1141, "X"=w1132) -> ("Filtered X"=w1140:dbl[])  [unwired: 8 in, 1 out]
                  n559 = Bundle By Name(cluster=w1132, "Y"=w1140) -> (w1131:waveform(dbl))
                }
                n560 = Bundle By Name(cluster=w1124, "data cut array"=w1123) -> (w1122:T11)
                n561 = property class="Clust (strict)"(reference=w1121, "Value"=w1122) -> ()  [unwired: 1 in, 2 out]
              }
            }
            n562 = property class="Bool (strict)"(reference=w1063) -> ("Value"=w1062:bool)  [unwired: 1 in, 2 out]
            n563 = Index Array(array=w1061, index="channel") -> (element=w1069:waveform(dbl))
            n564 = Decrement(x=w1035) -> (x-1=w1034:i32)
            n565 = Unbundle("singletonecontroll") -> ("advanced search"=w1057:cluster{"approx.freq.":dbl, "search(+/-%)":dbl}, "remove\ntone"=w1056:bool)
            n566 = case shown="True" "fit" {
              tunnel: w1053 -> [w1084 w1086]
              frame True {
                w1085 = u8 2 ("Z Scale.Scale Fit")
                n567 = property on="Property Node" class="IntGraph (strict)"(reference=w1084, "ZScale.ScaleFit"=w1085, "YScale.ScaleFit"=w1085, "XScale.ScaleFit"=w1085) -> ()  [unwired: 1 in, 2 out]
              }
              frame False {
                w1087 = u8 0 ("Z Scale.Scale Fit")
                n568 = property on="Property Node" class="IntGraph (strict)"(reference=w1086, "ZScale.ScaleFit"=w1087, "YScale.ScaleFit"=w1087, "XScale.ScaleFit"=w1087) -> ()  [unwired: 1 in, 2 out]
              }
            }
            n569 = property on="channel" class="Ring (strict)"("Strings []"=w1036, "Maximum"=w1034) -> ()  [unwired: 2 in, 2 out]
            n570 = case "singletone" shown="True" w1056 {
              tunnel: w1061 -> [_ w1094]
              tunnel: "export mode" -> [_ w1093]
              tunnel: w1057 -> [_ w1092]
              tunnel: w1060 -> [_ w1090]
              tunnel: w1044 -> [_ w1088]
              frame False {
              }
              frame True {
                n571 = for {
                  tunnel: w1094 -> [w1097] mode=indexing
                  tunnel: w1093 -> [w1099]
                  tunnel: w1092 -> [w1098]
                  tunnel: [w1095] -> w1089 mode=indexing
                  n572 = call-poly <vilib>:"Extract Single Tone Information.vi"("advanced search"=w1098, "export mode"=w1099, "time signal in"=w1097) -> ("exported signals"=w1096:T40)  [unwired: 3 in, 5 out]
                  n573 = Unbundle By Name(w1096) -> ("exported time signal"=w1095:waveform(dbl))
                }
                n574 = Bundle By Name(cluster=w1090, "data cut array"=w1089) -> (w1091:T11)
                n575 = property class="Clust (strict)"(reference=w1088, "Value"=w1091) -> ()  [unwired: 1 in, 2 out]
              }
            }
            n576 = case shown="True" w1062 {
              tunnel: w1069 -> [_ w1116]
              tunnel: w1057 -> [_ w1115]
              tunnel: "export mode" -> [_ w1114]
              tunnel: "color table" -> [_ w1110]
              tunnel: "freq.bins" -> [_ w1109]
              tunnel: "window info" -> [_ w1108]
              tunnel: "time-freq. sampling info" -> [_ w1107]
              tunnel: "spectrogam window info" -> [_ w1106]
              frame False {
              }
              frame True {
                n577 = call-poly <vilib>:"TFA STFT Spectrogram.vi"("window info"=w1106, "time-frequency sampling info"=w1107, "signal"=w1116) -> ("scale info"=w1117:variant, "spectrogram"=w1118:dbl[][])  [unwired: 6 in, 1 out]
                n578 = call-poly <vilib>:"Extract Single Tone Information.vi"("advanced search"=w1115, "export mode"=w1114, "time signal in"=w1116) -> ("detected phase (deg)"=w1111:dbl, "detected amplitude"=w1112:dbl, "detected frequency"=w1113:dbl, "exported signals"=w1101:T40)  [unwired: 3 in, 2 out]
                n579 = call-poly <vilib>:"TSA Welch.vi"("dB on? (T)"=FALSE, "frequency bins"=w1109, "window info"=w1108, "Xt"=w1116) -> ("PSD"=→"PSD":cluster{"f0":dbl, "df":dbl, "S(f)":dbl[]})  [unwired: 5 in, 2 out]
                n580 = Unbundle By Name(w1101) -> ("exported time signal"=→"singletoneresult":waveform(dbl))
                n581 = Bundle("detected frequency"=w1113, "detected amplitude"=w1112, "detected phase (deg)"=w1111) -> (→"singletone":T41)  [unwired: 1 in]
                n582 = control-ref of="Spectrogram"() -> (w1120:refnum<vi>)
                n583 = call-poly <vilib>:"TFA Configure Spectrogram Indicator.vi"("reference of TF spectrogram indicator"=w1120, "color table"=w1110, "dB on? (F)"="dB on?", "scale info"=w1117, "spectrogram"=w1118) -> ("TF spectrogram indicator"=→"Spectrogram":dbl[][])  [unwired: 2 in, 4 out]
              }
            }
          }
          frame 2 {
            w1142 = FALSE ("Visible")
            w1167 = FALSE ("Visible")
            w1170 = TRUE ("Visible")
            n584 = property class="Clust (strict)"(reference=w1187) -> ("Value"=w1186:T11)  [unwired: 1 in, 2 out]
            n585 = property class="Splitter"(reference=w1182, "Position"=25 ("Position:Top")) -> ()  [unwired: 1 in, 2 out]
            n586 = property class="Clust (strict)"(reference=w1143, "Visible"=w1142) -> ()  [unwired: 1 in, 2 out]
            n587 = property class="Clust (strict)"(reference=w1174, "Visible"=w1170, "Position"=T21 {"Left"=0, "Top"=0}) -> ()  [unwired: 1 in, 2 out]
            n588 = property class="TabCtl (strict)"(reference=w1188, "Visible"=w1167) -> ()  [unwired: 1 in, 2 out]
            n589 = property class="WFGraph (strict)"(reference=w1144, "Visible"=w1142) -> ()  [unwired: 1 in, 2 out]
            n590 = property class="WFGraph (strict)"(reference=w1145, "Visible"=w1167) -> ()  [unwired: 1 in, 2 out]
            n591 = property class="Clust (strict)"(reference=w1184, "Visible"=w1167) -> ()  [unwired: 1 in, 2 out]
            n592 = Unbundle By Name(w1186) -> ("data cut array"=w1181:waveform(dbl)[], "short data lables"=w1151:string[])
            n593 = Unbundle By Name("preproc.settings") -> ("maxFreqSet"=w1152:bool, "max.freq,Hz"=w1153:dbl, "FFT Window info.log/lin"=w1148:bool, "autoscale"=w1154:bool, "select1"=w1156:u16, "select2"=w1179:u16, "FFT Window info"=w1178:T42, "dist.,cm"=w1177:dbl, "PowerScale 2D"=w1176:dbl, "Plot.Line Width"=w1175:u8, "spectrogram\nsampling inf"=w1173:cluster{"time steps":i32, "frequency bins":i32}, "dB on?"=w1172:bool, "spctrgr.color"=w1171:u16, "spctrgrmWhich"=w1159:u16)
            n594 = Array Size(array=w1151) -> (size(s)=w1150:i32)
            n595 = case shown="False" w1154 {
              tunnel: w1153 -> [_ w1919]
              tunnel: w1152 -> [_ w1920]
              frame True {
                w1918 = u8 2 ("X Scale.Scale Fit")
                n596 = property on="Spectrogram" class="IntGraph (strict)"("XScale.ScaleFit"=w1918, "YScale.ScaleFit"=w1918, "ZScale.ScaleFit"=w1918) -> ()  [unwired: 2 in, 2 out]
                n597 = property on="frequency marginal integral" class="WFGraph (strict)"("XScale.ScaleFit"=w1918, "YScale.ScaleFit"=w1918) -> ()  [unwired: 2 in, 2 out]
                n598 = property on="instantaneous PSD" class="WFGraph (strict)"("XScale.ScaleFit"=w1918, "YScale.ScaleFit"=w1918) -> ()  [unwired: 2 in, 2 out]
                n599 = property on="time marginal integral" class="WFGraph (strict)"("XScale.ScaleFit"=w1918, "YScale.ScaleFit"=w1918) -> ()  [unwired: 2 in, 2 out]
              }
              frame False {
                n600 = case shown="False" w1920 {
                  tunnel: w1919 -> [w1921 _]
                  frame True {
                    w1922 = u8 0 ("X Scale.Scale Fit")
                    n601 = property on="Spectrogram" class="IntGraph (strict)"("XScale.ScaleFit"=w1922, "YScale.ScaleFit"=w1922, "ZScale.ScaleFit"=w1922, "YScale.Maximum"=w1921) -> ()  [unwired: 2 in, 2 out]
                    n602 = property on="frequency marginal integral" class="WFGraph (strict)"("XScale.ScaleFit"=w1922, "YScale.ScaleFit"=w1922, "XScale.Maximum"=w1921) -> ()  [unwired: 2 in, 2 out]
                    n603 = property on="instantaneous PSD" class="WFGraph (strict)"("XScale.ScaleFit"=w1922, "YScale.ScaleFit"=w1922, "XScale.Maximum"=w1921) -> ()  [unwired: 2 in, 2 out]
                    n604 = property on="time marginal integral" class="WFGraph (strict)"("XScale.ScaleFit"=w1922, "YScale.ScaleFit"=w1922) -> ()  [unwired: 2 in, 2 out]
                  }
                  frame False {
                    w1923 = u8 0 ("X Scale.Scale Fit")
                    n605 = property on="Spectrogram" class="IntGraph (strict)"("XScale.ScaleFit"=w1923, "YScale.ScaleFit"=w1923, "ZScale.ScaleFit"=w1923) -> ()  [unwired: 2 in, 2 out]
                    n606 = property on="frequency marginal integral" class="WFGraph (strict)"("XScale.ScaleFit"=w1923, "YScale.ScaleFit"=w1923) -> ()  [unwired: 2 in, 2 out]
                    n607 = property on="instantaneous PSD" class="WFGraph (strict)"("XScale.ScaleFit"=w1923, "YScale.ScaleFit"=w1923) -> ()  [unwired: 2 in, 2 out]
                    n608 = property on="time marginal integral" class="WFGraph (strict)"("XScale.ScaleFit"=w1923, "YScale.ScaleFit"=w1923) -> ()  [unwired: 2 in, 2 out]
                  }
                }
              }
            }
            n609 = case shown="False" w1148 {
              frame True {
                w1916 = u8 1 ("Y Scale.Mapping Mode")
                n610 = property on="instantaneous PSD" class="WFGraph (strict)"("YScale.Mapping Mode"=w1916) -> ()  [unwired: 2 in, 2 out]
                n611 = property on="frequency marginal integral" class="WFGraph (strict)"("YScale.Mapping Mode"=w1916) -> ()  [unwired: 2 in, 2 out]
                n612 = property on="time marginal integral" class="WFGraph (strict)"("YScale.Mapping Mode"=w1916) -> ()  [unwired: 2 in, 2 out]
                n613 = property on="cut.filtered" class="WFGraph (strict)"("YScale.Mapping Mode"=w1916) -> ()  [unwired: 2 in, 2 out]
              }
              frame False {
                w1917 = u8 0 ("Y Scale.Mapping Mode")
                n614 = property on="instantaneous PSD" class="WFGraph (strict)"("YScale.Mapping Mode"=w1917) -> ()  [unwired: 2 in, 2 out]
                n615 = property on="frequency marginal integral" class="WFGraph (strict)"("YScale.Mapping Mode"=w1917) -> ()  [unwired: 2 in, 2 out]
                n616 = property on="time marginal integral" class="WFGraph (strict)"("YScale.Mapping Mode"=w1917) -> ()  [unwired: 2 in, 2 out]
                n617 = property on="cut.filtered" class="WFGraph (strict)"("YScale.Mapping Mode"=w1917) -> ()  [unwired: 2 in, 2 out]
              }
            }
            n618 = control-ref of="Spectrogram"() -> (w1155:refnum<vi>)
            n619 = control-ref of="spctrgrmWhich"() -> (w1168:refnum<vi>)
            n620 = Index Array(array=w1151, index=w1159) -> (element=w1160:string)
            n621 = Decrement(x=w1150) -> (x-1=w1149:i32)
            n622 = control-ref of="select2"() -> (w1162:refnum<vi>)
            n623 = property class="IntGraph (strict)"(reference=w1155, "Caption.Text"=w1160) -> ()  [unwired: 1 in, 2 out]
            n624 = property class="Ring (strict)"(reference=w1168, "Strings []"=w1151, "Maximum"=w1149) -> (reference out=w1158:refnum<vi>)  [unwired: 1 in, 1 out]
            n625 = case shown="0, Default" w1156 {
              tunnel: w1185 -> [w1931 w1939 w1946]
              tunnel: [w1929 w1937 w1945] -> w1166
              tunnel: w1157 -> [w1928 w1936 w1947]
              tunnel: w1170 -> [w1925 w1932 w1943]
              tunnel: FALSE ("Visible") -> [w1924 w1933 w1942]
              tunnel: [w1927 w1935 w1940] -> w1165
              tunnel: w1162 -> [w1926 w1934 w1944]
              frame 0, Default {
                n626 = property class="WFGraph (strict)"(reference=w1931, "Visible"=w1925) -> (reference out=w1930:refnum<vi>)  [unwired: 1 in, 1 out]
                n627 = property class="Ring (strict)"(reference=w1926, "Visible"=w1924) -> ()  [unwired: 1 in, 2 out]
                n628 = property class="Clust (strict)"(reference=w1928, "Visible"=w1924) -> (reference out=w1927:refnum<vi>)  [unwired: 1 in, 1 out]
                n629 = invoke on="Invoke Node" class="WFGraph (strict)" method="FitControlToPane"(reference=w1930) -> (reference out=w1929:refnum<vi>)  [unwired: 2 in, 2 out]
              }
              frame 1 {
                n630 = property class="WFGraph (strict)"(reference=w1939, "Visible"=w1932) -> (reference out=w1938:refnum<vi>)  [unwired: 1 in, 1 out]
                n631 = property class="Ring (strict)"(reference=w1934, "Visible"=w1932) -> ()  [unwired: 1 in, 2 out]
                n632 = property class="Clust (strict)"(reference=w1936, "Visible"=w1933) -> (reference out=w1935:refnum<vi>)  [unwired: 1 in, 1 out]
                n633 = invoke on="Invoke Node" class="WFGraph (strict)" method="FitControlToPane"(reference=w1938) -> (reference out=w1937:refnum<vi>)  [unwired: 2 in, 2 out]
              }
              frame 3 {
                n634 = property class="WFGraph (strict)"(reference=w1946, "Visible"=w1942) -> (reference out=w1945:refnum<vi>)  [unwired: 1 in, 1 out]
                n635 = property class="Ring (strict)"(reference=w1944, "Visible"=w1942) -> ()  [unwired: 1 in, 2 out]
                n636 = property class="Clust (strict)"(reference=w1947, "Visible"=w1943, "Position"=T21 {"Left"=0, "Top"=0}) -> (reference out=w1940:refnum<vi>)  [unwired: 1 in, 1 out]
              }
            }
            n637 = property on="Property Node" class="Ring (strict)"(reference=w1158, "DecKeyBind"=T24 {"Focus"=FALSE, "Control"=FALSE, "Shift"=FALSE, "Key"="<PageDown>"} ("Decrement Key Binding"), "IncKeyBind"=T24 {"Focus"=FALSE, "Control"=FALSE, "Shift"=FALSE, "Key"="<PageUp>"} ("Decrement Key Binding")) -> ()  [unwired: 1 in, 2 out]
            n638 = flat-sequence {
              tunnel: w1181 -> [w1203]
              tunnel: w1179 -> [w1202]
              tunnel: w1178 -> [w1201]
              tunnel: w1177 -> [w1200]
              tunnel: w1176 -> [w1199]
              tunnel: w1175 -> [w1198]
              tunnel: w1173 -> [w1196]
              tunnel: w1172 -> [w1195]
              tunnel: w1171 -> [w1194]
              tunnel: w1166 -> [w1193]
              tunnel: w1165 -> [w1192]
              tunnel: w1156 -> [w1189]
              tunnel: w1151 -> [w1191]
              tunnel: [w1190] -> w1147
              tunnel: [w1189] -> w1146
              tunnel: w1147 -> [w1892]
              tunnel: w1146 -> [w1891]
              frame #0 {
                n639 = control-ref of="return pressed?"() -> (w1204:refnum<vi>)
                n640 = property class="Bool (strict)"(reference=w1204) -> ("Value"=w1197:bool)  [unwired: 1 in, 2 out]
                n641 = control-ref of="Spectrogram"() -> (w1190:refnum<vi>)
                n642 = case shown="True" w1197 {
                  tunnel: w1191 -> [_ w1220]
                  tunnel: w1203 -> [_ w1219]
                  tunnel: w1189 -> [_ w1218]
                  tunnel: w1202 -> [_ w1217]
                  tunnel: w1201 -> [_ w1216]
                  tunnel: w1200 -> [_ w1215]
                  tunnel: w1199 -> [_ w1214]
                  tunnel: w1198 -> [_ w1213]
                  tunnel: w1196 -> [_ w1212]
                  tunnel: w1195 -> [_ w1211]
                  tunnel: w1194 -> [_ w1210]
                  tunnel: w1191 -> [_ w1209]
                  tunnel: w1193 -> [_ w1208]
                  tunnel: w1192 -> [_ _]
                  tunnel: w1190 -> [_ w1205]
                  frame False {
                  }
                  frame True {
                    w1206 = u8 2 ("X Scale.Scale Fit")
                    n643 = property class="WFGraph (strict)"(reference=w1208, "XScale.ScaleFit"=w1206, "YScale.ScaleFit"=w1206) -> (reference out=w1207:refnum<vi>)  [unwired: 1 in, 1 out]
                    n644 = case shown="0, Default" w1218 {
                      tunnel: w1220 -> [w1229 w1260 w1690 _]
                      tunnel: w1219 -> [w1223 w1266 w1694 w1877]
                      tunnel: w1213 -> [w1228 w1246 w1681 _]
                      tunnel: w1217 -> [_ w1242 _ _]
                      tunnel: w1216 -> [_ w1245 w1680 w1875]
                      tunnel: w1214 -> [_ w1244 w1679 _]
                      tunnel: w1215 -> [_ w1243 _ _]
                      tunnel: w1212 -> [_ _ _ w1874]
                      tunnel: w1211 -> [_ _ _ w1873]
                      tunnel: w1210 -> [_ _ _ w1872]
                      tunnel: w1209 -> [_ _ _ _]
                      tunnel: w1207 -> [w1224 w1239 w1675 _]
                      tunnel: w1205 -> [_ _ _ w1867]
                      frame 0, Default {
                        n645 = property class="WFGraph (strict)"(reference=w1224, "Value"=w1223) -> (reference out=w1225:refnum<vi>)  [unwired: 1 in, 1 out]
                        n646 = for {
                          N -> [w1233]
                          tunnel: w1225 -> [w1238]
                          tunnel: w1229 -> [w1236] mode=indexing
                          tunnel: w1228 -> [w1235]
                          tunnel: [w1234] -> w1227
                          tunnel: [w1233] -> w1226
                          i -> [w1237]
                          n647 = property class="WFGraph (strict)"(reference=w1238, "Active Plot"=w1237, "Plot.Plot Name"=w1236, "Plot.Line Width"=w1235) -> (reference out=w1234:refnum<vi>)  [unwired: 1 in, 1 out]
                        }
                        n648 = In Range and Coerce(upper limit=20, x=w1226, lower limit=1) -> (coerced(x)=w1230:i32)  [unwired: 1 out]
                        n649 = property class="WFGraph (strict)"(reference=w1227, "LegNumRows"=w1230, "LegPlotMin"=w1226, "XScale.NameLbl.Text"="time, s" ("X Scale.Name Label.Text"), "YScale.NameLbl.Text"="amplitude, a.u." ("Y Scale.Name Label.Text")) -> ()  [unwired: 1 in, 2 out]
                      }
                      frame 1 {
                        n650 = case shown="0, Default" w1242 {
                          tunnel: ["_coh" "_crspsd" "_phase" "_phasedegr" "_wavenum"] -> w1241
                          tunnel: w1239 -> [w1268 w1270 w1273 w1276 w1279]
                          frame 0, Default {
                            n651 = property class="WFGraph (strict)"(reference=w1268, "YScale.NameLbl.Text"="a.u." ("Y Scale.Name Label.Text")) -> ()  [unwired: 1 in, 2 out]
                          }
                          frame 1 {
                            n652 = property class="WFGraph (strict)"(reference=w1270, "YScale.NameLbl.Text"="power, a.u." ("Y Scale.Name Label.Text")) -> ()  [unwired: 1 in, 2 out]
                          }
                          frame 2 {
                            n653 = property class="WFGraph (strict)"(reference=w1273, "YScale.NameLbl.Text"="rad" ("Y Scale.Name Label.Text")) -> ()  [unwired: 1 in, 2 out]
                          }
                          frame 3 {
                            n654 = property class="WFGraph (strict)"(reference=w1276, "YScale.NameLbl.Text"="degree" ("Y Scale.Name Label.Text")) -> ()  [unwired: 1 in, 2 out]
                          }
                          frame 4 {
                            n655 = property class="WFGraph (strict)"(reference=w1279, "YScale.NameLbl.Text"="cm^-1" ("Y Scale.Name Label.Text")) -> ()  [unwired: 1 in, 2 out]
                          }
                        }
                        n656 = Unbundle By Name(w1245) -> ("Length"=w1262:i32, "Overlap (%)"=w1263:dbl)  [unwired: 1 out]
                        n657 = Array Size(array=w1266) -> (size(s)=w1265:i32)
                        n658 = Decrement(x=w1265) -> (x-1=w1264:i32)
                        n659 = To Double Precision Float(number=w1262) -> (double precision float=w1261:dbl)
                        n660 = for {
                          N: w1264 -> [w1320]
                          tunnel: w1266 -> [w1317]
                          tunnel: w1263 -> [w1316]
                          tunnel: w1261 -> [w1315]
                          tunnel: w1244 -> [w1314]
                          tunnel: w1243 -> [w1313]
                          tunnel: w1260 -> [w1311]
                          tunnel: [w1309] -> w1258 mode=concatenating
                          tunnel: [w1308] -> w1257 mode=concatenating
                          tunnel: [w1307] -> w1256 mode=concatenating
                          tunnel: [w1306] -> w1255 mode=concatenating
                          tunnel: [w1305] -> w1254 mode=concatenating
                          tunnel: [w1304] -> w1259 mode=concatenating
                          tunnel: w1241 -> [w1303]
                          i -> [w1312]
                          n661 = Subtract(x=w1320, y=w1312) -> (x-y=w1319:i32)
                          n662 = Index Array(array=w1311, index=w1312) -> (element=w1310:string)
                          n663 = Index Array(array=w1317, index=w1312) -> (element=w1318:waveform(dbl))
                          n664 = for {
                            N: w1319 -> [_]
                            tunnel: w1318 -> [w1348]
                            tunnel: w1317 -> [w1352]
                            tunnel: w1312 -> [w1351]
                            tunnel: w1316 -> [w1344]
                            tunnel: w1315 -> [w1343]
                            tunnel: w1314 -> [w1342]
                            tunnel: w1313 -> [w1341]
                            tunnel: w1311 -> [w1338]
                            tunnel: w1310 -> [w1335]
                            tunnel: [w1331] -> w1309 mode=indexing
                            tunnel: [w1325] -> w1308 mode=indexing
                            tunnel: [w1324] -> w1307 mode=indexing
                            tunnel: [w1323] -> w1306 mode=indexing
                            tunnel: [w1322] -> w1305 mode=indexing
                            tunnel: [w1333] -> w1304 mode=indexing
                            tunnel: w1303 -> [w1321]
                            i -> [w1349]
                            n665 = Increment(x=w1351) -> (x+1=w1350:i32)
                            n666 = Add(x=w1350, y=w1349) -> (x+y=w1337:i32)
                            n667 = Unbundle By Name(w1348) -> ("Y"=w1347:dbl[], "dt"=w1340:dbl)
                            n668 = Index Array(array=w1352, index=w1337) -> (element=w1346:waveform(dbl))
                            n669 = Index Array(array=w1338, index=w1337) -> (element=w1334:string)
                            n670 = Reciprocal(x=w1340) -> (1/x=w1339:dbl)
                            n671 = Unbundle By Name(w1346) -> ("Y"=w1345:dbl[])
                            n672 = mathscript code="noverlap = fftsize *(overl_per/100);\nwindow = win_hamming(fftsize);\nwin=win_hamming(fftsize);\nflag = 'none';\n%PSD================================\n%[Pxx, f] = psd_welch(X, win, noverlap, fftsize, fs);\n%[Pyy, f] = psd_welch(Y, win, noverlap, fftsize, fs);\n%Pxx=Pxx*PowerScale\n%Pyy=Pyy*PowerScale\n\n\n[Rxy, f] = coherence(X,Y, fftsize, fs, window, noverlap,flag);\ndf = f(2)-f(1);\nffirst=f(1);\n%==================================\n%crossPhase-wavenum\nSxy1= crosspsd(X, Y,  win, noverlap, fftsize, fs)\nSxy=conjugate(Sxy1)*PowerScale\n%SxyReshape =reshapemx(Sxy,size(Sxy,2),1);\nimagSxy=imag(Sxy);\nrealSxy=real(Sxy);\n\n%phaseSxy = atan2(imagSxy,realSxy);\nphaseSxy = angle(Sxy) %!!! the same as \"atan2\"\nwavenumXY = angle(Sxy)/probedist;\n\nphaseSxyDegrees = rad_to_deg(phaseSxy)\nunwrapSxy = unwrapphase(phaseSxy, pi, 1)\n%unwrapphaseSxy=reshapemx(unwrapSxy,size(Sxy,2),1)\nabsSxy=abs(Sxy)"("X"=w1347, "Y"=w1345, "fftsize"=w1343, "fs"=w1339, "overl_per"=w1344, "probedist"=w1341, "PowerScale"=w1342) -> ("Rxy"=w1332:dbl[], "wavenumXY"=w1329:dbl[], "phaseSxy"=w1327:dbl[], "phaseSxyDegrees"=w1326:dbl[], "absSxy"=w1328:dbl[], "df"=w1330:dbl)  [unwired: 3 out]
                            n673 = Concatenate Strings(w1335, "*AND*" ("string"), w1334, w1321) -> (w1333:string)
                            n674 = Bundle By Name "phaseDegrees"("dt"=w1330, "Y"=w1326) -> (w1323:waveform(dbl))  [unwired: 1 in]
                            n675 = Bundle By Name "wavenum"("dt"=w1330, "Y"=w1329) -> (w1322:waveform(dbl))  [unwired: 1 in]
                            n676 = Bundle By Name "crosspsd"("dt"=w1330, "Y"=w1328) -> (w1325:waveform(dbl))  [unwired: 1 in]
                            n677 = Bundle By Name "coher"("dt"=w1330, "Y"=w1332) -> (w1331:waveform(dbl))  [unwired: 1 in]
                            n678 = Bundle By Name "phase"("dt"=w1330, "Y"=w1327) -> (w1324:waveform(dbl))  [unwired: 1 in]
                          }
                        }
                        n679 = control-ref of="cut.filtered"() -> (w1253:refnum<vi>)
                        n680 = case shown="0, Default" w1242 {
                          tunnel: w1258 -> [w1284 _ _ _ _]
                          tunnel: w1257 -> [_ w1287 _ _ _]
                          tunnel: w1256 -> [_ _ w1290 _ _]
                          tunnel: w1255 -> [_ _ _ w1293 _]
                          tunnel: w1254 -> [_ _ _ _ w1296]
                          tunnel: w1253 -> [w1283 w1286 w1289 w1292 w1295]
                          tunnel: [w1282 w1285 w1288 w1291 w1294] -> w1252
                          frame 0, Default {
                            n681 = property class="WFGraph (strict)"(reference=w1283, "Value"=w1284) -> (reference out=w1282:refnum<vi>)  [unwired: 1 in, 1 out]
                          }
                          frame 1 {
                            n682 = property class="WFGraph (strict)"(reference=w1286, "Value"=w1287) -> (reference out=w1285:refnum<vi>)  [unwired: 1 in, 1 out]
                          }
                          frame 2 {
                            n683 = property class="WFGraph (strict)"(reference=w1289, "Value"=w1290) -> (reference out=w1288:refnum<vi>)  [unwired: 1 in, 1 out]
                          }
                          frame 3 {
                            n684 = property class="WFGraph (strict)"(reference=w1292, "Value"=w1293) -> (reference out=w1291:refnum<vi>)  [unwired: 1 in, 1 out]
                          }
                          frame 4 {
                            n685 = property class="WFGraph (strict)"(reference=w1295, "Value"=w1296) -> (reference out=w1294:refnum<vi>)  [unwired: 1 in, 1 out]
                          }
                        }
                        n686 = for {
                          N -> [w1298]
                          tunnel: w1259 -> [w1300] mode=indexing
                          tunnel: w1252 -> [w1302]
                          tunnel: [w1299] -> w1251
                          tunnel: [w1298] -> w1247
                          tunnel: w1246 -> [w1297]
                          i -> [w1301]
                          n687 = property class="WFGraph (strict)"(reference=w1302, "Active Plot"=w1301, "Plot.Plot Name"=w1300, "Plot.Line Width"=w1297) -> (reference out=w1299:refnum<vi>)  [unwired: 1 in, 1 out]
                        }
                        n688 = In Range and Coerce(upper limit=20, x=w1247, lower limit=0) -> (coerced(x)=w1248:i32)  [unwired: 1 out]
                        n689 = property class="WFGraph (strict)"(reference=w1251, "LegNumRows"=w1248, "LegPlotMin"=w1247, "XScale.NameLbl.Text"="frequency, Hz" ("X Scale.Name Label.Text")) -> ()  [unwired: 1 in, 2 out]
                      }
                      frame 2 {
                        n690 = Unbundle By Name(w1680) -> ("Length"=w1692:i32, "Overlap (%)"=w1693:dbl)  [unwired: 1 out]
                        n691 = Array Size(array=w1694) -> (size(s)=w1678:i32)
                        n692 = To Double Precision Float(number=w1692) -> (double precision float=w1691:dbl)
                        n693 = for {
                          N: w1678 -> [_]
                          tunnel: w1694 -> [w1703]
                          tunnel: w1693 -> [w1716]
                          tunnel: w1691 -> [w1715]
                          tunnel: w1679 -> [w1714]
                          tunnel: w1690 -> [w1712]
                          tunnel: [w1710] -> w1688 mode=indexing
                          tunnel: [w1709] -> w1689 mode=indexing
                          i -> [w1713]
                          n694 = Index Array(array=w1703, index=w1713) -> (element=w1717:waveform(dbl))
                          n695 = Unbundle By Name(w1717) -> ("Y"=w1708:dbl[], "dt"=w1707:dbl)
                          n696 = Index Array(array=w1712, index=w1713) -> (element=w1711:string)
                          n697 = Reciprocal(x=w1707) -> (1/x=w1706:dbl)
                          n698 = mathscript code="noverlap = fftsize *(overl_per/100);\nwindow = win_hamming(fftsize);\nwin=win_hamming(fftsize);\n%flag = 'none';\n%PSD================================\n[Pxx, f] = psd_welch(X, win, noverlap, fftsize, fs);\n%[Pyy, f] = psd_welch(Y, win, noverlap, fftsize, fs);\nPxx=Pxx*PowerScale\n%Pyy=Pyy*PowerScale\n\n\n%[Rxy, f] = coherence(X,Y, fftsize, fs, window, noverlap,flag);\ndf = f(2)-f(1);\n%ffirst=f(1);\n%==================================\n%crossPhase-wavenum\n%Sxy1= crosspsd(X, Y,  win, noverlap, fftsize, fs)\n%Sxy=conjugate(Sxy1)*PowerScale\n%SxyReshape =reshapemx(Sxy,size(Sxy,2),1);\n%imagSxy=imag(Sxy);\n%realSxy=real(Sxy);\n\n%phaseSxy = atan2(imagSxy,realSxy);\n%phaseSxy = angle(Sxy) %!!! the same as \"atan2\"\n%wavenumXY = angle(Sxy)/probedist;\n\n%phaseSxyDegrees = rad_to_deg(phaseSxy)\n%unwrapSxy = unwrapphase(phaseSxy, pi, 1)\n%unwrapphaseSxy=reshapemx(unwrapSxy,size(Sxy,2),1)\n%absSxy=abs(Sxy)"("X"=w1708, "fftsize"=w1715, "fs"=w1706, "overl_per"=w1716, "PowerScale"=w1714) -> ("df"=w1704:dbl, "Pxx"=w1705:dbl[])  [unwired: 2 out]
                          n699 = Concatenate Strings(w1711, "_" ("string"), "PSD" ("string")) -> (w1709:string)
                          n700 = Bundle By Name "psd"("dt"=w1704, "Y"=w1705) -> (w1710:waveform(dbl))  [unwired: 1 in]
                        }
                        n701 = property class="WFGraph (strict)"(reference=w1675, "YScale.NameLbl.Text"="power, a.u." ("Y Scale.Name Label.Text")) -> ()  [unwired: 1 in, 2 out]
                        n702 = property class="WFGraph (strict)"(reference=w1675, "Value"=w1688) -> (reference out=w1687:refnum<vi>)  [unwired: 1 in, 1 out]
                        n703 = for {
                          N -> [w1696]
                          tunnel: w1689 -> [w1698] mode=indexing
                          tunnel: w1687 -> [w1700]
                          tunnel: [w1697] -> w1686
                          tunnel: [w1696] -> w1682
                          tunnel: w1681 -> [w1695]
                          i -> [w1699]
                          n704 = property class="WFGraph (strict)"(reference=w1700, "Active Plot"=w1699, "Plot.Plot Name"=w1698, "Plot.Line Width"=w1695) -> (reference out=w1697:refnum<vi>)  [unwired: 1 in, 1 out]
                        }
                        n705 = In Range and Coerce(upper limit=20, x=w1682, lower limit=0) -> (coerced(x)=w1683:i32)  [unwired: 1 out]
                        n706 = property class="WFGraph (strict)"(reference=w1686, "LegNumRows"=w1683, "LegPlotMin"=w1682, "XScale.NameLbl.Text"="frequency, Hz" ("X Scale.Name Label.Text")) -> ()  [unwired: 1 in, 2 out]
                      }
                      frame 3 {
                        n707 = Array Size(array=w1877) -> (size(s)=w1876:i32)
                        n708 = Unbundle By Name(w1875) -> ("Window"=w1871:u16, "Length"=w1870:i32)
                        n709 = for {
                          N: w1876 -> [_]
                          tunnel: w1877 -> [w1889]
                          tunnel: w1874 -> [w1887]
                          tunnel: w1873 -> [w1884]
                          tunnel: w1872 -> [w1883]
                          tunnel: [w1882] -> w1869 mode=indexing
                          tunnel: w1871 -> [w1881]
                          tunnel: w1870 -> [w1880]
                          tunnel: w1867 -> [w1879]
                          tunnel: [w1878] -> w1868
                          i -> [w1890]
                          n710 = Bundle("Window"=w1881, "Length"=w1880) -> (w1888:cluster{"Window":u16, "Length":i32})  [unwired: 1 in]
                          n711 = Index Array(array=w1889, index=w1890) -> (element=w1886:waveform(dbl))
                          n712 = call-poly <vilib>:"TFA STFT Spectrogram.vi"("window info"=w1888, "time-frequency sampling info"=w1887, "signal"=w1886) -> ("scale info"=w1878:variant, "spectrogram"=w1885:dbl[][])  [unwired: 6 in, 1 out]
                          n713 = call-poly <vilib>:"TFA Configure Spectrogram Indicator.vi"("reference of TF spectrogram indicator"=w1879, "color table"=w1883, "dB on? (F)"=w1884, "scale info"=w1878, "spectrogram"=w1885) -> ("TF spectrogram indicator"=w1882:dbl[][])  [unwired: 2 in, 4 out]
                        }
                        "spectrogram array" <- w1869
                        "scale info" <- w1868
                      }
                    }
                  }
                }
              }
              frame #1 {
                n714 = case shown="3" w1891 {
                  tunnel: w1892 -> [_ w1894]
                  frame 0, Default {
                  }
                  frame 3 {
                    n715 = control-ref of="scale info"() -> (w1904:refnum<vi>)
                    n716 = property class="LVVar"(reference=w1904) -> ("Value"=w1908:variant)  [unwired: 1 in, 2 out]
                    n717 = property class="IntGraph (strict)"(reference=w1894, "Active Cursor"=u32 0) -> ("Cursor.Cursor X"=w1893:dbl)  [unwired: 1 in, 2 out]
                    n718 = call <vilib>:"TFA Get Time and Freq Scale Info.vi"("scale info"=w1908) -> ("frequency info"=w1910:T43, "time info"=w1909:T44)  [unwired: 8 in, 1 out]
                    n719 = Unbundle By Name(w1909) -> ("time offset"=w1900:dbl, "time multiplier"=w1902:dbl)
                    n720 = control-ref of="spectrogram array"() -> (w1897:refnum<vi>)
                    n721 = control-ref of="spctrgrmWhich"() -> (w1895:refnum<vi>)
                    n722 = property class="Ring (strict)"(reference=w1895) -> ("Value"=w1896:u16)  [unwired: 1 in, 2 out]
                    n723 = property class="Arr (strict)"(reference=w1897) -> ("Value"=w1898:dbl[][][])  [unwired: 1 in, 2 out]
                    n724 = Subtract(x=w1893, y=w1900) -> (x-y=w1901:dbl)
                    n725 = Divide(x=w1901, y=w1902) -> (x/y=w1903:dbl)
                    n726 = Index Array(array=w1898, index (dim 0)=w1896) -> (element=w1911:dbl[][])  [unwired: 2 in]
                    n727 = Unbundle By Name(w1910) -> ("frequency offset"=w1905:dbl, "frequency multiplier"=w1906:dbl)
                    n728 = Index Array(array=w1911, index (row)=w1903) -> (element=w1907:dbl[])  [unwired: 1 in]
                    n729 = call <vilib>:"TFA Marginal Integration.vi"("scale info"=w1908, "spectrogram"=w1911) -> ("time marginal integral"=w1913:cluster{"t0":dbl, "dt":dbl, "power":dbl[]}, "frequency marginal integral"=w1912:cluster{"f0":dbl, "df":dbl, "spectrum":dbl[]})  [unwired: 7 in, 1 out]
                    n730 = Bundle("frequency offset"=w1905, "frequency multiplier"=w1906, "Value"=w1907) -> (w1914:T45)  [unwired: 1 in]
                    n731 = Bundle("time info"=w1909, "frequency info"=w1910, "Value"=w1911, "frequency marginal integral"=w1912, "time marginal integral"=w1913, w1914, "Cursor.Cursor X"=w1893) -> (→"spctrgrmClaster":T46)  [unwired: 1 in]
                  }
                }
              }
            }
          }
          frame 3 {
            w1970 = TRUE ("Visible")
            w2004 = FALSE ("Visible")
            n732 = property class="Splitter"(reference=w2008, "Position"=25 ("Splitter Position")) -> ()  [unwired: 1 in, 2 out]
            n733 = property class="Clust (strict)"(reference=w1971, "Visible"=w1970, "Position"=T21 {"Left"=10, "Top"=10} ("Position 2")) -> ()  [unwired: 1 in, 2 out]
            n734 = property class="Clust (strict)"(reference=w2010, "Visible"=w2004) -> ()  [unwired: 1 in, 2 out]
            n735 = property class="TabCtl (strict)"(reference=w2003, "Visible"=w2004) -> ()  [unwired: 1 in, 2 out]
            n736 = property class="WFGraph (strict)"(reference=w2002, "Visible"=w1970) -> (reference out=w2001:refnum<vi>)  [unwired: 1 in, 1 out]
            n737 = property class="WFGraph (strict)"(reference=w2006, "Visible"=w2004) -> ()  [unwired: 1 in, 2 out]
            n738 = property class="Clust (strict)"(reference=w2005, "Visible"=w2004) -> ()  [unwired: 1 in, 2 out]
            n739 = property class="WFGraph (strict)"(reference=w2007, "Visible"=w2004) -> ()  [unwired: 1 in, 2 out]
            n740 = property class="Clust (strict)"(reference=w1999) -> ("Value"=w2000:T11)  [unwired: 1 in, 2 out]
            n741 = invoke class="WFGraph (strict)" method="FitControlToPane"(reference=w2001) -> ()  [unwired: 2 in, 3 out]
            n742 = Unbundle By Name(w2000) -> ("data cut array"=w1952:waveform(dbl)[], "short data lables"=w1998:string[])
            n743 = property on="Isat" class="Ring (strict)"("Strings []"=w1998) -> ()  [unwired: 2 in, 2 out]
            n744 = property on="Vfl" class="Ring (strict)"("Strings []"=w1998) -> ()  [unwired: 2 in, 2 out]
            n745 = property on="V+" class="Ring (strict)"("Strings []"=w1998) -> ()  [unwired: 2 in, 2 out]
            n746 = Unbundle By Name("tripleProbeSetting") -> ("Isat"=w1982:u16, "Vfl"=w1981:u16, "V+"=w1980:u16, "a=1/ln2"=w1977:dbl, "Vfl*"=w1975:dbl, "[V+]*"=w1976:dbl, "Te*"=w1974:dbl, "/Rn(ohm)"=w1979:dbl, "/amplif"=w1978:dbl, "Spr, cm^2"=w1972:dbl, "plasma, a.m.u"=w1973:dbl, "Ne*10^x"=w1966:dbl)
            n747 = property on="data info template" class="Clust (strict)"() -> ("Value"=w1954:T1)  [unwired: 2 in, 2 out]
            n748 = Array Size(array=w1952) -> (size(s)=w1951:i32)
            n749 = Index Array "Isat,V"(array=w1952, index=w1982) -> (element=w1964:waveform(dbl))
            n750 = Index Array "V+"(array=w1952, index=w1980) -> (element=w1962:waveform(dbl))
            n751 = Index Array "Vfl"(array=w1952, index=w1981) -> (element=w1963:waveform(dbl))
            n752 = Index Array(array=w1952) -> (element=w1956:waveform(dbl))  [unwired: 1 in]
            n753 = Divide "Isat,V"(x=w1964, y=w1979) -> (x/y=w1995:waveform(dbl))
            n754 = Multiply "V+, V"(x=w1962, y=w1976) -> (x*y=w1957:waveform(dbl))
            n755 = Multiply "Vfl, V"(x=w1963, y=w1975) -> (x*y=w1958:waveform(dbl))
            n756 = Get Waveform Attribute(5:w1954, 6:"info" ("name"), 7:w1956) -> (1:w1953:T1)  [unwired: 1 in, 3 out]
            n757 = Subtract(1:w1958, 2:w1957) -> (0:w1997:waveform(dbl))  [unwired: 1 in, 1 out]
            n758 = Divide(x=w1995, y=w1978) -> (x/y=w1994:waveform(dbl))
            n759 = Unbundle By Name(w1953) -> ("channels_in_file"=w1949:i32)
            n760 = Multiply "Te, eV"(x=w1977, y=w1997) -> (x*y=w1985:waveform(dbl))
            n761 = Divide(x=w1951, y=w1949) -> (x/y=w1950:dbl)
            n762 = Multiply "Isat, mA"(x=w1994, y=1000.0) -> (x*y=w1959:waveform(dbl))
            n763 = Multiply(x=w1985, y=w1974) -> (x*y=w1996:waveform(dbl))
            n764 = Reciprocal(x=w1973) -> (1/x=w1992:dbl)
            n765 = Add(1:w1958, 2:w1996) -> (0:w1984:waveform(dbl))  [unwired: 1 in, 1 out]
            n766 = Square Root(x=w1985) -> (sqrt(x)=w1990:waveform(dbl))
            n767 = Square Root(x=w1992) -> (sqrt(x)=w1991:dbl)
            n768 = for {
              N: w1950 -> [_]
              tunnel: w1949 -> [w2014]
              shift-right: [w2013] -> _
              shift-left: 0 -> [w2012]
              n769 = Add(x=w2014, y=w2012) -> (x+y=w2013:i32)
              n770 = Wait (ms)(milliseconds to wait=u32 500) -> ()  [unwired: 1 out]
            }
            n771 = Divide(1:w1990, 2:w1959) -> (0:w1988:waveform(dbl))  [unwired: 1 in, 1 out]
            n772 = Multiply(x=w1972, y=w1991) -> (x*y=w1989:dbl)
            n773 = Divide(x=w1988, y=w1989) -> (x/y=w1987:waveform(dbl))
            n774 = for {
              N: w1966 -> [_]
              shift-right: [w2016] -> w1965
              shift-left: 1.0 -> [w2017]
              n775 = Multiply(x=10.0, y=w2017) -> (x*y=w2016:dbl)
            }
            n776 = Multiply(x=9000000000.0, y=w1987) -> (x*y=w1969:waveform(dbl))
            n777 = Divide(x=w1969, y=w1965) -> (x/y=w1968:waveform(dbl))
            n778 = Build Array(w1985, w1984, w1968, w1959, w1958, w1957) -> (→"triple probe":waveform(dbl)[])
          }
        }
      }
    }
  }
